vi "Auto_New.vi"() -> ()   [LabVIEW 2023]
uses:
  Control/Saurabh/prosucer_consumer_enum.ctl
  <vilib>/addons/database/NI_Database_API.lvlib
  Global/Global 1.vi
  Global/DATA LOG.vi
  <vilib>/Utility/error.llb/DialogType.ctl
  <vilib>/addons/database/Connection.llb/DB Tools Open Connec (String).vi
panel:
  out "SHIFT":string
  in  "BARCODE RECIPE":string(combo)
  out "PLC COM.":bool
  out "SHIFT_DATA":string[](array[string])
  out "OP40 BARCODE STRING EMPRTY":bool
  out "OP30 BARCODE STRING EMPRTY":bool
  out "stop":bool
  out "error out 2":errorcluster
  out "Shift 4":i32
  out "Time Stamp Out":timestamp[](array[timestamp]) format="%<%X>T"
  out "Time Stamp Out 4":timestamp[](array[timestamp]) format="%<%X>T"
  out "Shift_change":bool
  out "appended array":string[][](array[string])
  out "SHIFT_DATA 2":string[](array[string])
  in  "error in (no error)":errorcluster
  in  "Tab Control":enum32{"Screen 1", "Screen 2"}(tab)
  out "OP 50":bool
  out "OP 40":bool
  out "OP 30":bool
  out "OP - 50":T1
  out "OP - 40":T2
  out "OP - 30":T3
  in  "stop 2":bool
  out "OP - 10":T4
  in  "SIMULATE INPUT":bool[](array[boolean])=[FALSE, FALSE, FALSE, FALSE]
  out "OP - 20":T5
  out "OP 10 & 20":bool
  out "OP - 110":cluster{"BARCODE":string}
  out "OP - 80":T6
  out "OP - 70":T7
  out "OP - 90":T8
  out "OP - 100":T9
  out "OP - 60":T10
  out "OP 60":bool
  out "OP 70 & 80":bool
  out "OP 90 -100 - 110":bool
  # "SENSOR MIN VLTG"
  # "Op10 20\nOp30\nOp 40\nOp50\nOp60\nOp70-80\nOp 90-100-110"
  # "OP - 50"
  # "OP - 40"
  # "OP - 30"
  # "OP - 10"
  # "OP - 20"
  # "Op10 20\nOp30\nOp 40\nOp50\nOp60\nOp70-80\nOp 90-100-110"
  # "OP - 110"
  # "OP - 80"
  # "OP - 70"
  # "OP - 90"
  # "OP - 100"
  # "OP - 60"
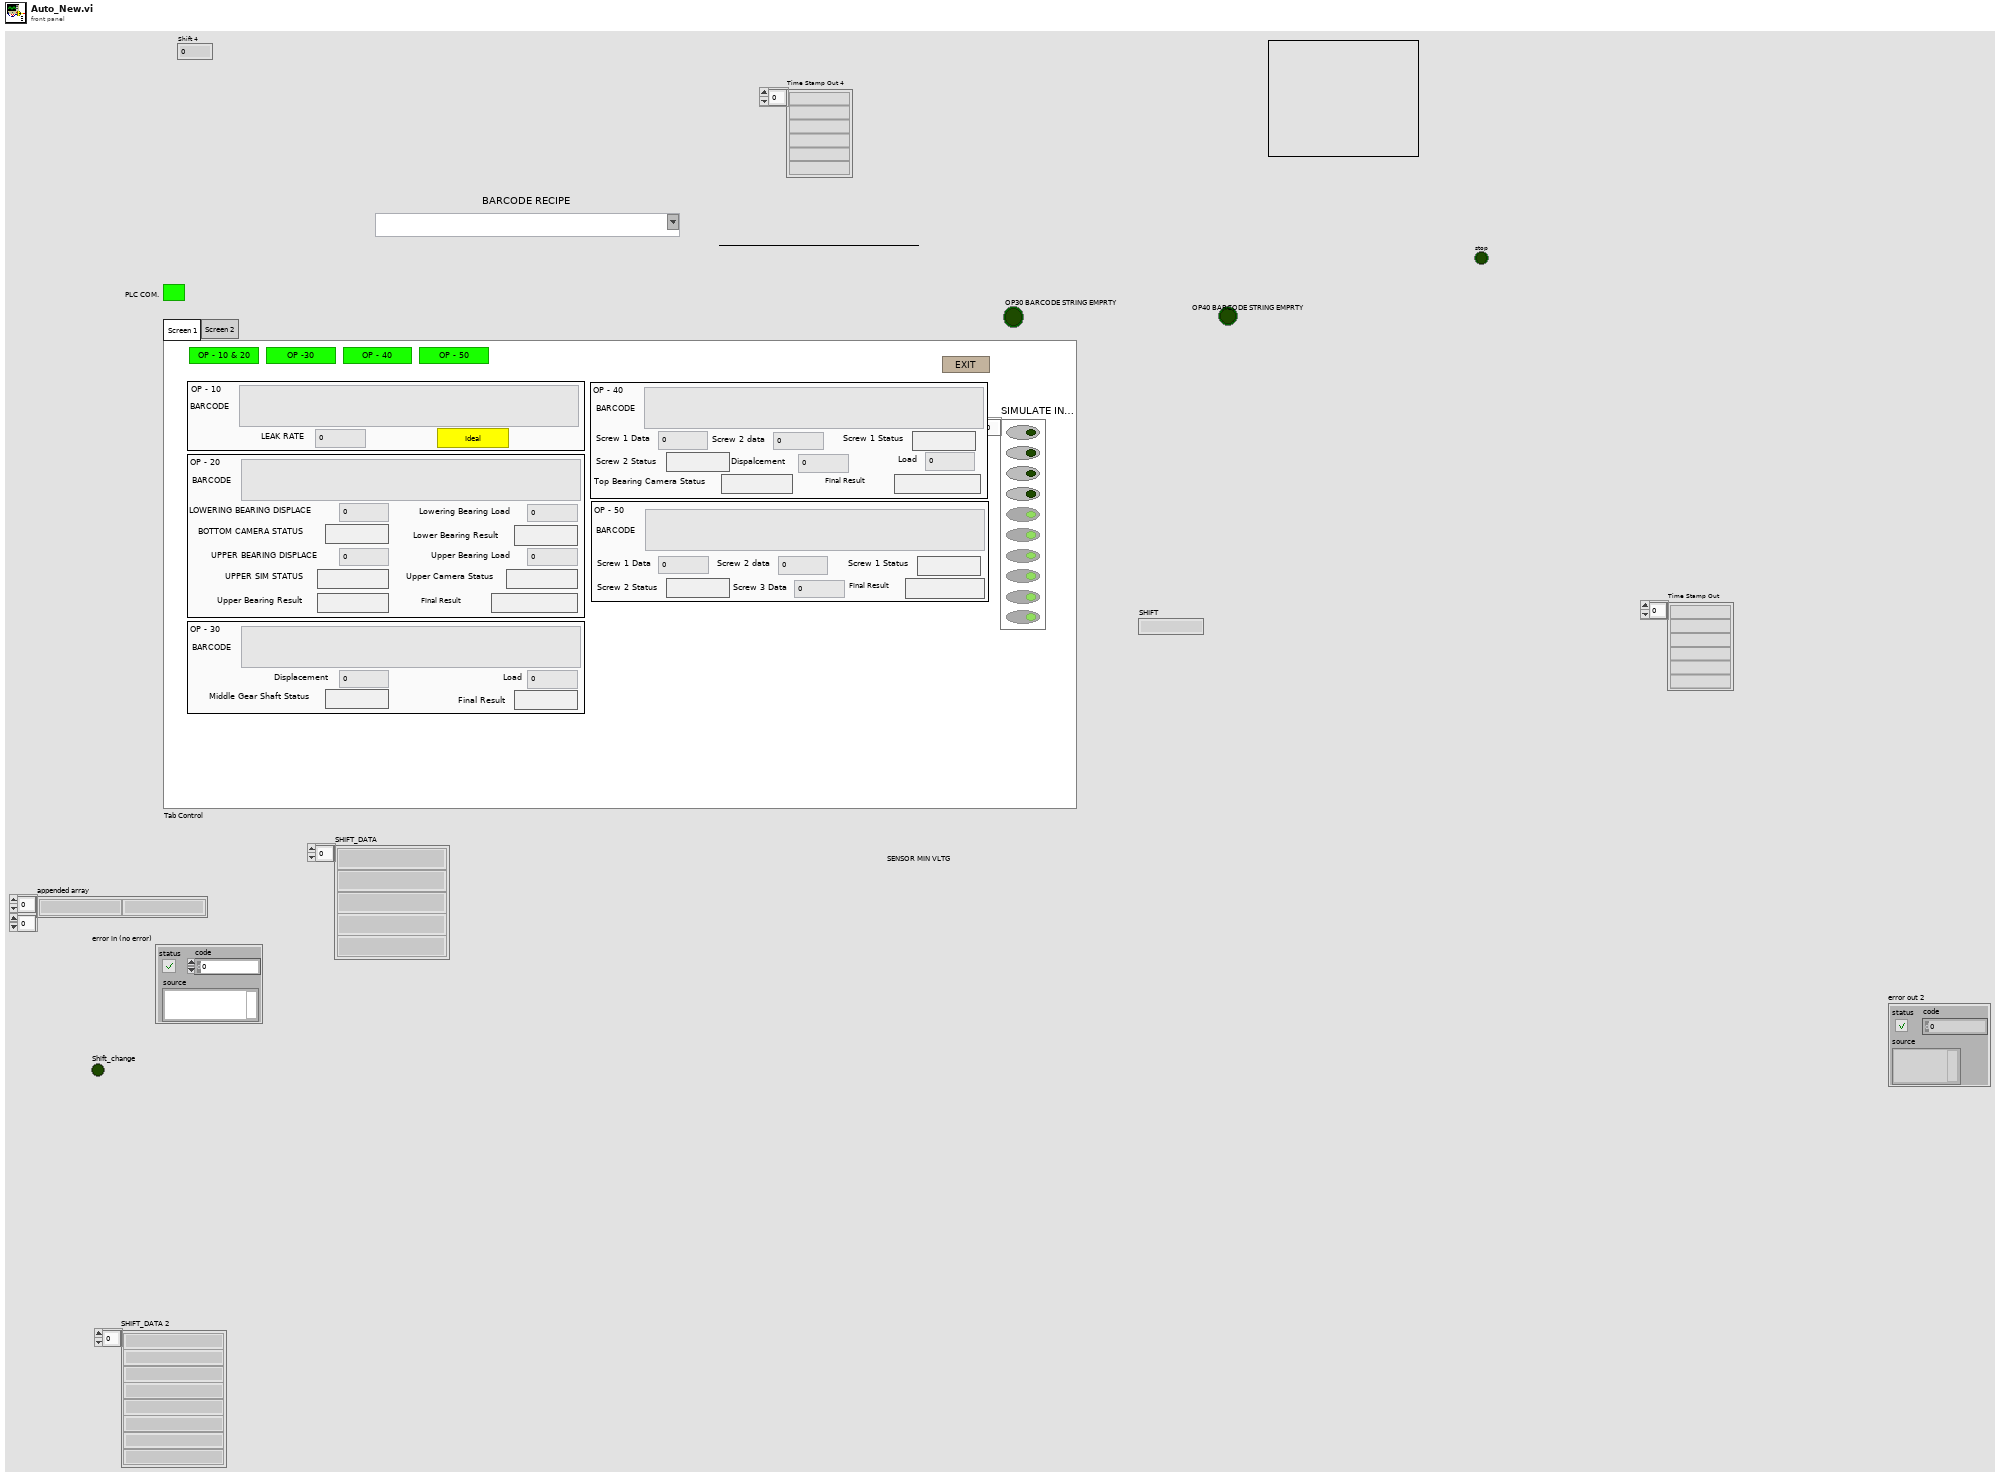
[diagram p1: front panel]
types:
  T1 = cluster{"BARCODE":string, "Screw 1 Data":dbl, "Screw 2 data":dbl, "Screw 1 Status":bool, "Screw 2 Status":bool, "Screw 3 Data":dbl, "Final Result":bool}
  T2 = cluster{"BARCODE":string, "Screw 1 Data":dbl, "Screw 2 data":dbl, "Screw 1 Status":bool, "Screw 2 Status":bool, "Dispalcement ":dbl, "Load ":dbl, "Top Bearing Camera Status":bool, "Final Result":bool}
  T3 = cluster{"BARCODE":string, "Displacement":dbl, "Load":dbl, "Middle Gear Shaft Status":bool, "Final Result":bool}
  T4 = cluster{"BARCODE":string, "LEAK RATE":dbl, "RESULT":bool}
  T5 = cluster{"BARCODE":string, "LOWERING BEARING DISPLACE":dbl, "Lowering Bearing Load":dbl, "BOTTOM CAMERA STATUS":bool, "Lower Bearing Result":bool, "UPPER BEARING DISPLACE":dbl, "Upper Bearing Load ":dbl, "UPPER SIM STATUS":bool, "Upper Camera Status":bool, "Upper Bearing Result":bool, "Final Result":bool}
  T6 = cluster{"BARCODE":string, "Load":dbl, "Final Result":bool, "Dispensing":bool}
  T7 = cluster{"BARCODE":string, "Sensor MIN Vltg":dbl, "Sensor MAX Vltg":dbl, "Final Result":bool}
  T8 = cluster{"BARCODE":string, "Seat LT Data":dbl, "Seat Status":bool, "Steam LT Data":dbl, "Final Result":bool}
  T9 = cluster{"BARCODE":string, "Sensor O/P Open V":dbl, "Start Of Close Sensor V":dbl, "Final Result":bool, "Sensor O/P Full Close V":dbl, "Response Time FWD (mSec)":dbl, "Response Time REV (mSec)":dbl, "Motor V Start Of Close A":dbl, "Motor V Full Close B R":dbl, "Motor V Start Back C":dbl, "Motor V Full Open D":dbl, "Motor RMS Current A":dbl}
  T10 = cluster{"BARCODE":string, "Screw 1 Data":dbl, "Screw 2 data":dbl, "Screw 1 Status":bool, "Screw 2 Status":bool, "Screw3 Data":dbl, "Final Result":bool, "Screw3 Status":bool, "Screw4 Data":dbl, "Screw5 Data":dbl, "Screw4 Status":bool, "Screw5 Status":bool, "Screw6 Data":dbl, "Screw6 Status":bool}
  T11 = cluster{"OP - 10":cluster{"BARCODE":string, "LEAK RATE":dbl, "RESULT":bool}, "OP - 20":cluster{"BARCODE":string, "LOWERING BEARING DISPLACE":dbl, "LOWERING BEARING LOAD":dbl, "BOTTOM CAMERA STATUS":bool, "LOWER BEARING RESULT":bool, "UPPER BEARING DISPLACE":dbl, "UPPER BEARING LOAD ":dbl, "UPPER SIM STATUS":bool, "UPPER CAMERA STATUS":bool, "UPPER BEARING RESULT":bool, "FINAL RESULT":bool}, "OP - 30":cluster{"BARCODE":string, "Displacement":dbl, "Load":dbl, "Middle Gear Shaft Status":bool, "Final Result":bool}, "OP - 40":cluster{"BARCODE":string, "Screw 1 Data":dbl, "Screw 2 data":dbl, "Screw 1 Status":bool, "Screw 2 Status":bool, "Dispalcement ":dbl, "Load ":dbl, "Top Bearing Camera Status":bool, "Final Result":bool}, "OP - 50":cluster{"BARCODE":string, "Screw 1 Data":dbl, "Screw 2 data":dbl, "Screw 1 Status":bool, "Screw 2 Status":bool, "Screw 3 Data":dbl, "Final Result":bool}, "OP - 60":cluster{"BARCODE":string, "Screw 1 Data":dbl, "Screw 2 data":dbl, "Screw 1 Status":bool, "Screw 2 Status":bool, "Screw3 Data":dbl, "Final Result":bool, "Screw3 Status":bool, "Screw4 Data":dbl, "Screw5 Data":dbl, "Screw4 Status":bool, "Screw5 Status":bool, "Screw6 Data":dbl, "Screw6 Status":bool}, "OP - 70":cluster{"BARCODE":string, "Sensor MIN Vltg":dbl, "Sensor MAX Vltg":dbl, "Final Result":bool}, "OP - 80":cluster{"BARCODE":string, "Load":dbl, "Final Result":bool, "Dispensing":bool}, "OP - 90":cluster{"BARCODE":string, "Seat LT Data":dbl, "Seat Status":bool, "Steam LT Data":dbl, "Final Result":bool}, "OP - 100":cluster{"BARCODE":string, "Sensor O/P Open V":dbl, "Start Of Close Sensor V":dbl, "Final Result":bool, "Sensor O/P Full Close V":dbl, "Response Time FWD (mSec)":dbl, "Response Time REV (mSec)":dbl, "Motor V Start Of Close A":dbl, "Motor V Full Close B R":dbl, "Motor V Start Back C":dbl, "Motor V Full Open D":dbl, "Motor RMS Current A":dbl}, "OP - 110":cluster{"BARCODE":string}}
  T12 = typedef "prosucer_consumer_enum.ctl" = enum16{"SCAN1", "SCAN2", "SCAN3", "SCAN4", "SCAN5", "SCAN6", "SCAN7", "SCAN8", "SCAN9", "SCAN10", "SCAN11", "STOP", "DATALOG1", "DATALOG2", "DATALOG3", "DATALOG4", "DATALOG5", "DATALOG6", "DATALOG7", "DATALOG8", "DATALOG9", "DATALOG10", "DATALOG11", "-1", "CYCLE_START1", "CYCLE_START2", "CYCLE_START3", "CYCLE_START4", "BARCODE RECIPE", "EMERGENCY STOP"}
  T13 = typedef "NI_Database_API.lvlib/Conn ObjectReference.ctl" = refnum<k1>
  T14 = typedef "DialogType.ctl" = u16
  T15 = cluster{"trimmed string":string, "SHIFT":string, "date/time string":string, string, "Input 2":string}
  T16 = cluster{"SHIFT":string, "date/time string":string, "Input 2":string}
  T17 = cluster{"Input 2":string, "Input 2":string, "Input 2":string, "Input 2":string, "Input 2":string, "Input 2":string, "Input 2":string, "Input 2":string, "Input 2":string, "Input 2":string}
  T18 = cluster{"SHIFT":string, "date/time string":string, void}
  T19 = cluster{"BARCODE":string, "LOWERING BEARING DISPLACE":dbl, "LOWERING BEARING LOAD":dbl, "BOTTOM CAMERA STATUS":bool, "LOWER BEARING RESULT":bool, "UPPER BEARING DISPLACE":dbl, "UPPER BEARING LOAD ":dbl, "UPPER SIM STATUS":bool, "UPPER CAMERA STATUS":bool, "UPPER BEARING RESULT":bool, "FINAL RESULT":bool}
  T20 = enum32{"invalid app kind", "Development System", "Run Time System", "Student Edition", "Embedded LabVIEW", "Evaluation", "Custom"}
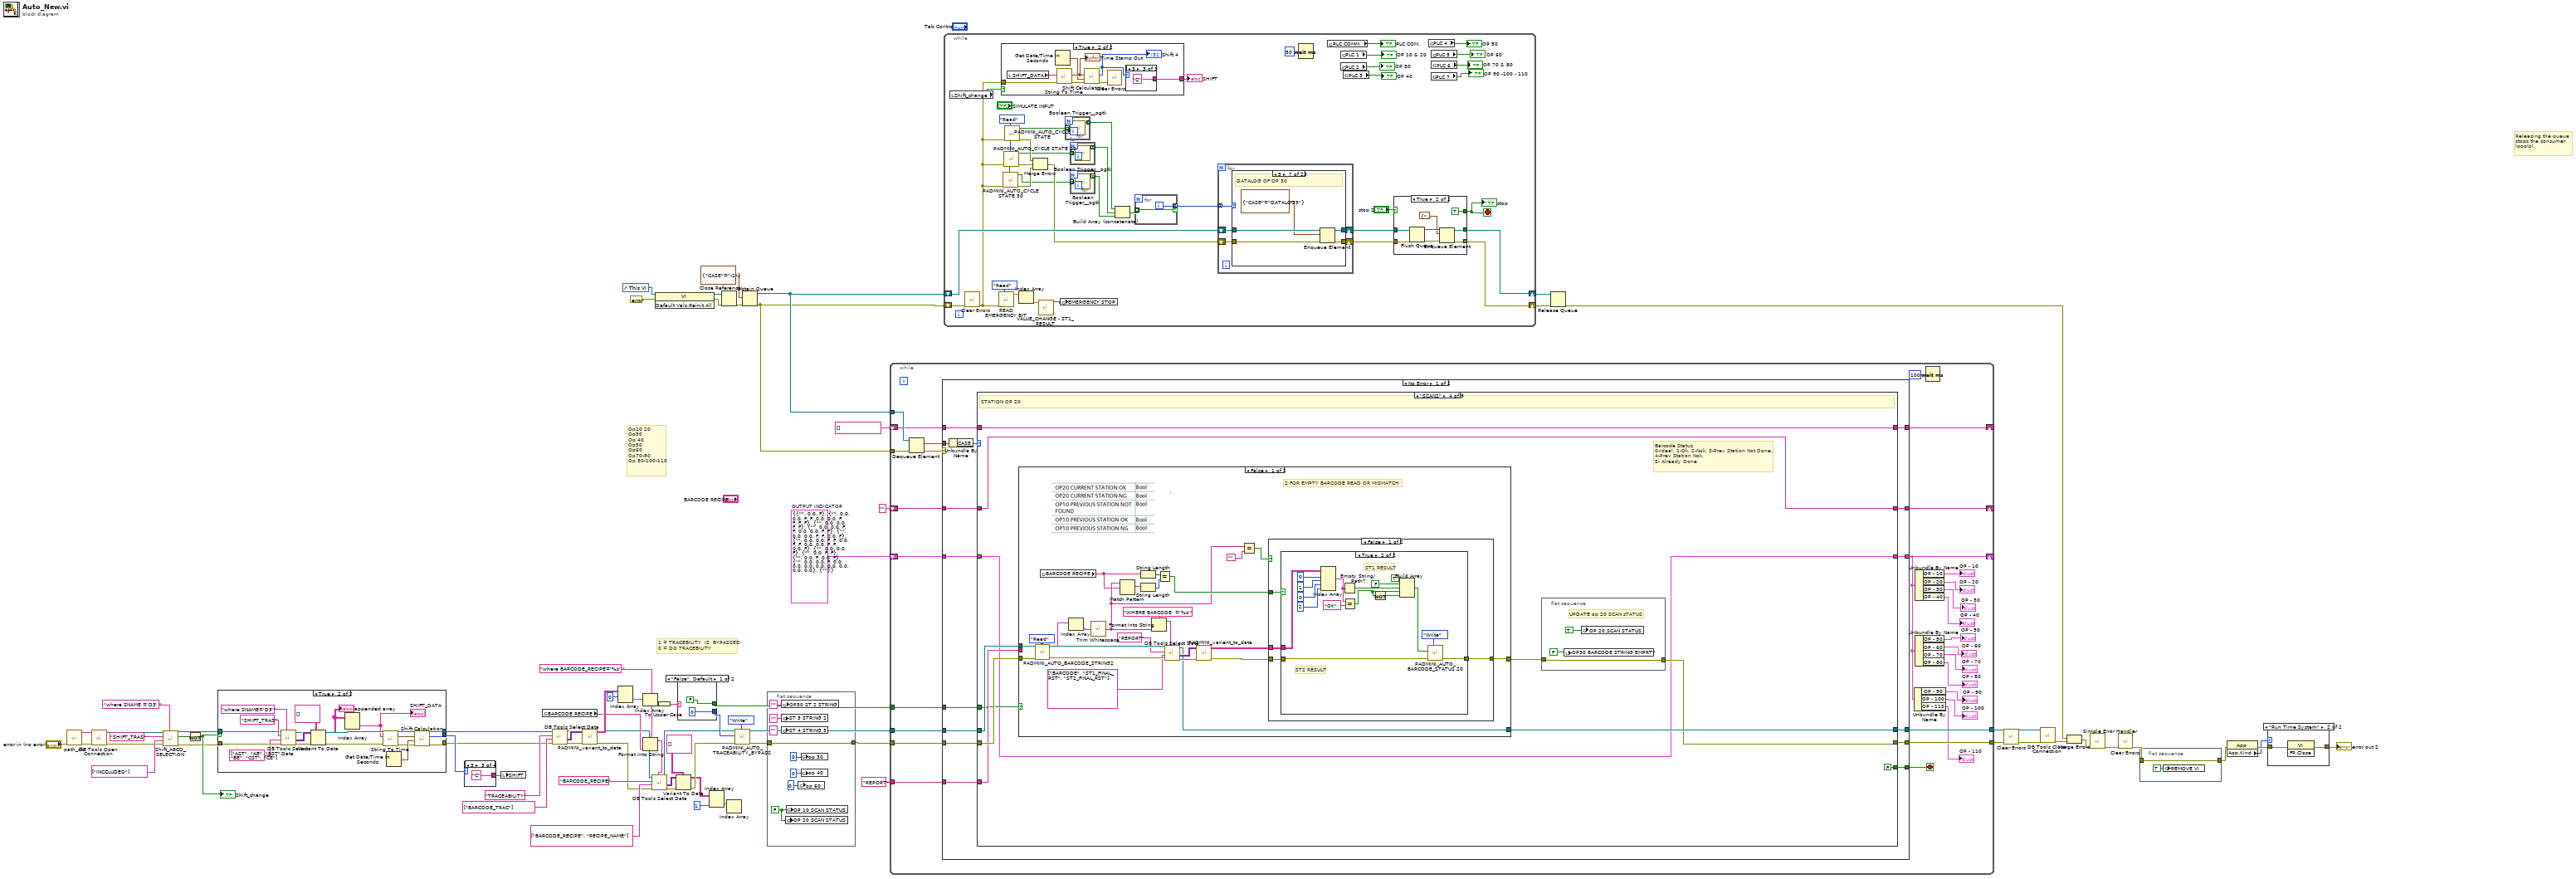
[diagram p0: block diagram]
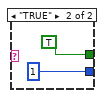
[diagram p2: hidden frame]
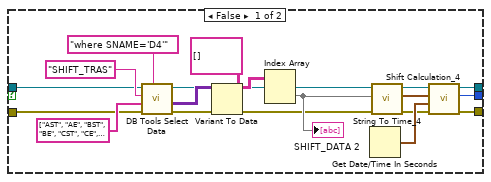
[diagram p3: hidden frame]
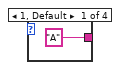
[diagram p4: hidden frame]
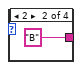
[diagram p5: hidden frame]
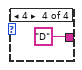
[diagram p6: hidden frame]
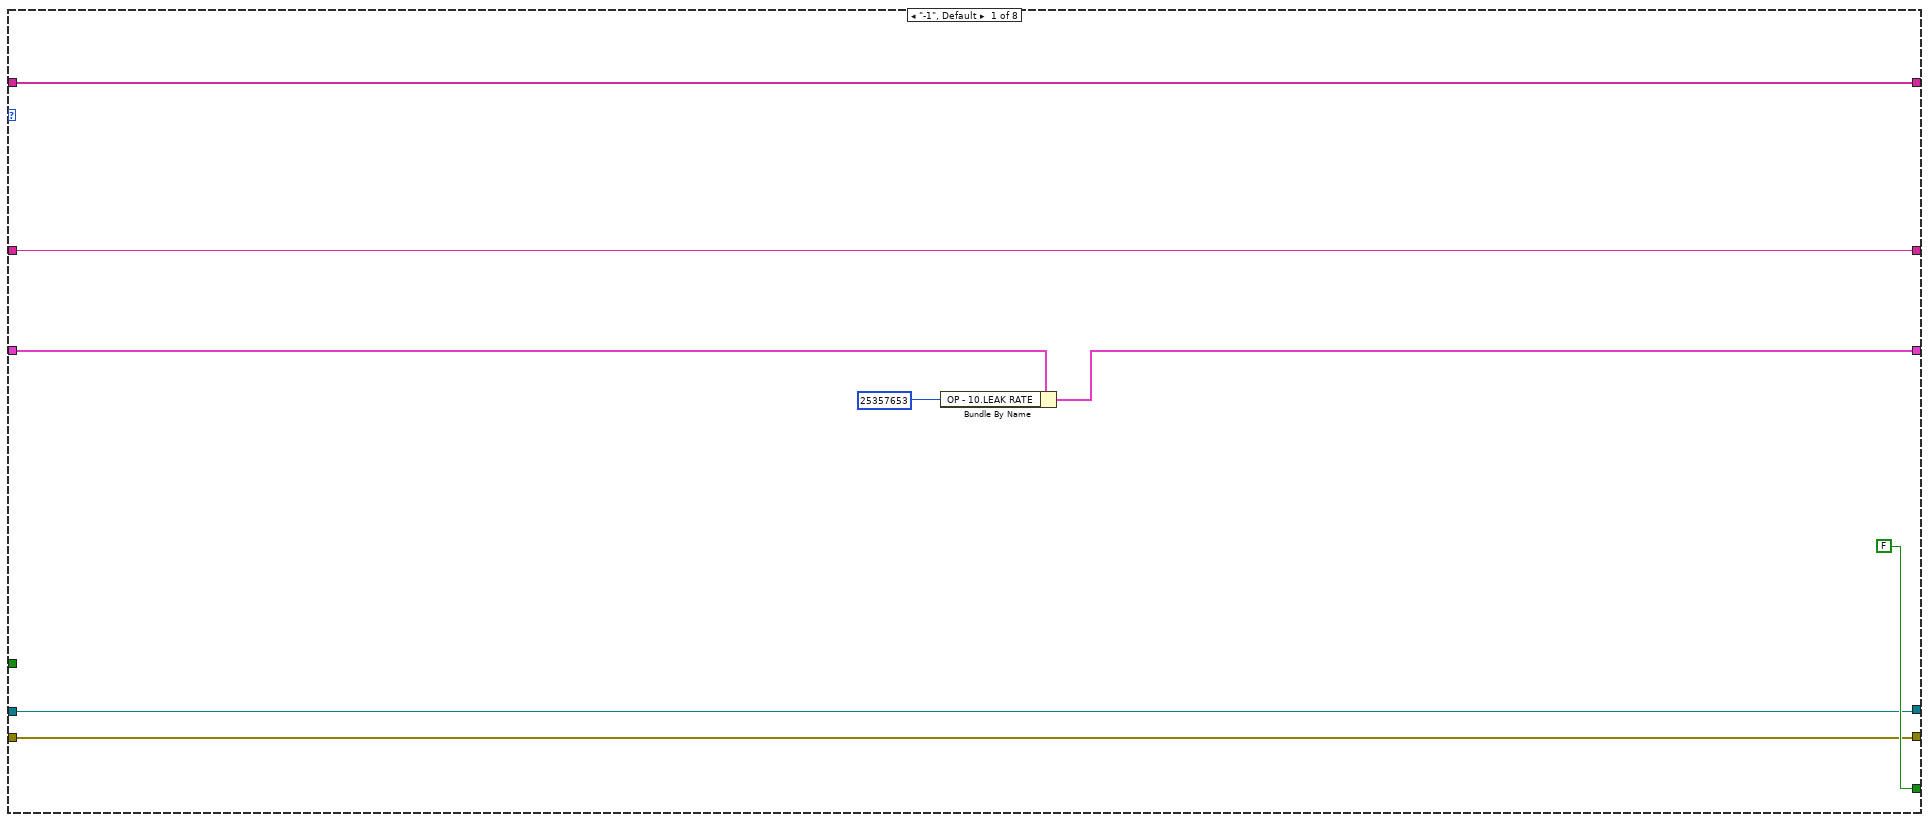
[diagram p7: hidden frame]
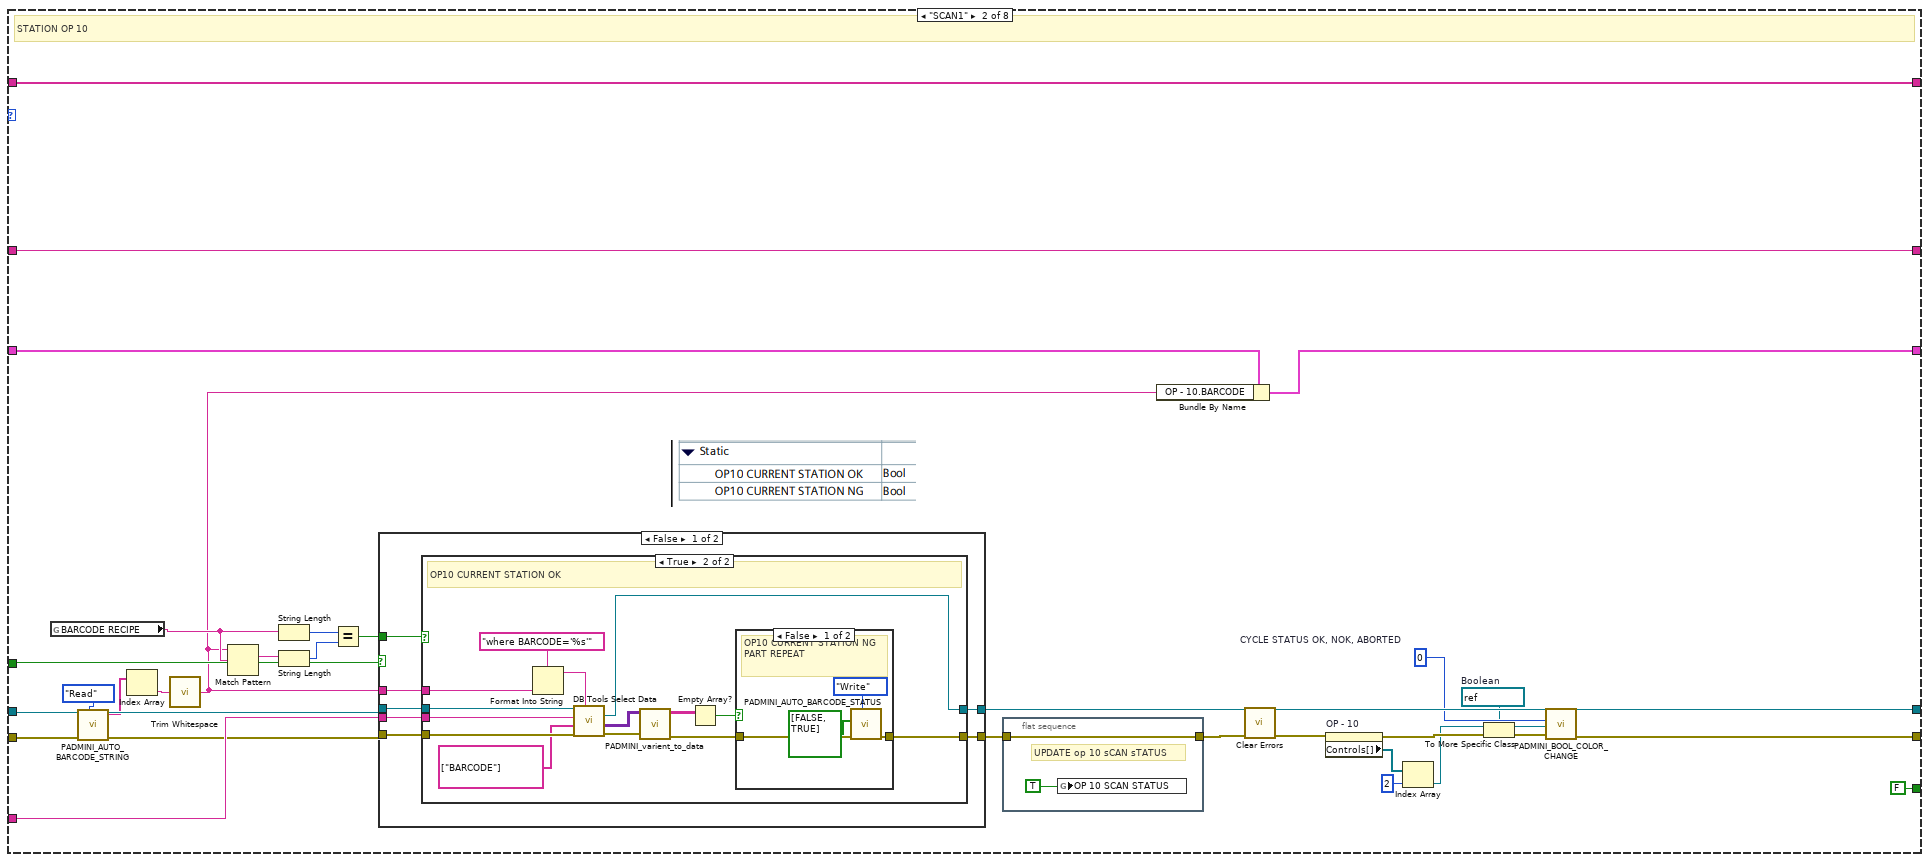
[diagram p8: hidden frame]
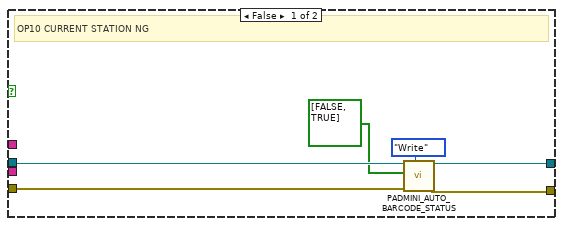
[diagram p9: hidden frame]
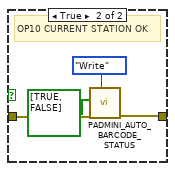
[diagram p10: hidden frame]
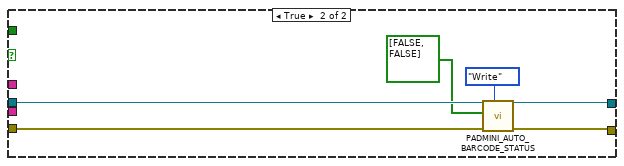
[diagram p11: hidden frame]
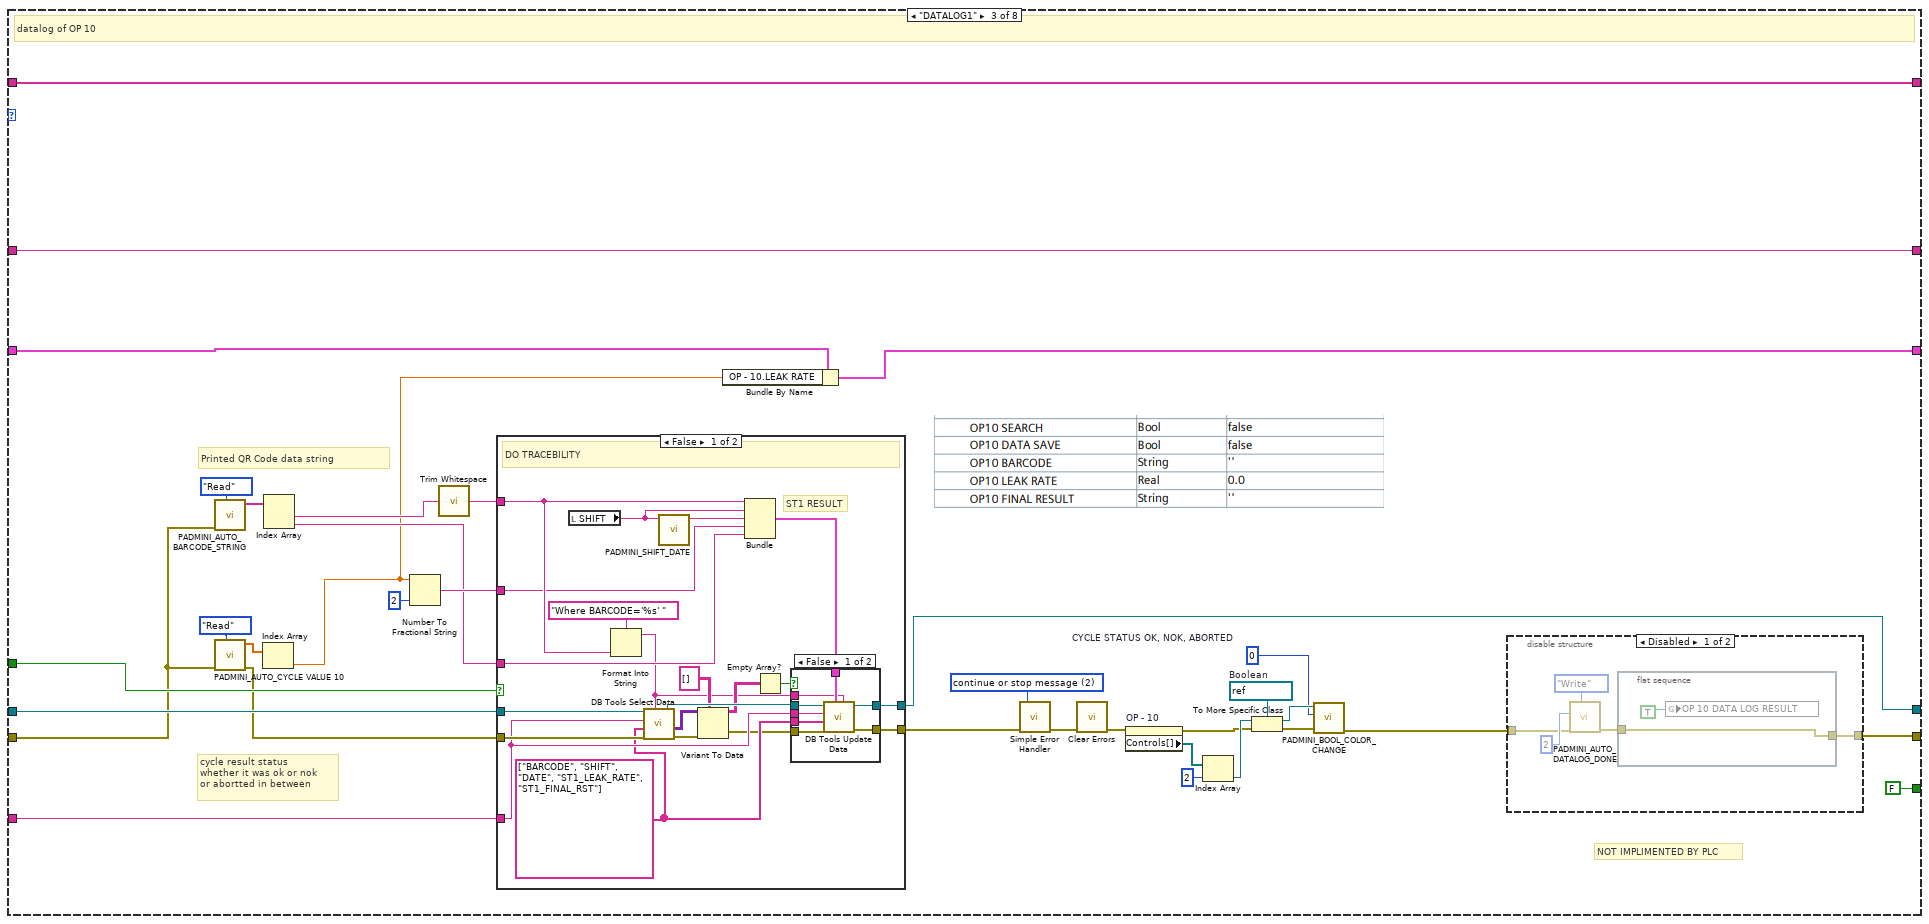
[diagram p12: hidden frame]
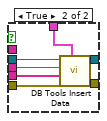
[diagram p14: hidden frame]
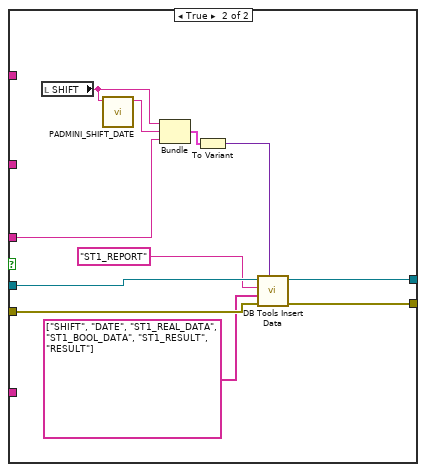
[diagram p15: hidden frame]
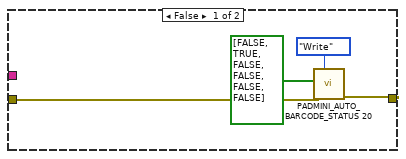
[diagram p16: hidden frame]
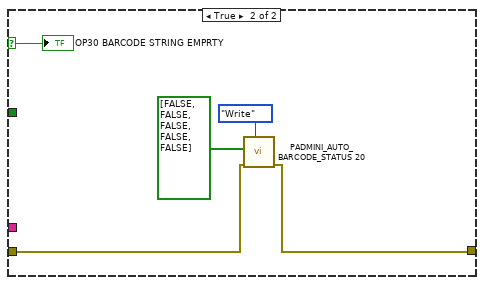
[diagram p17: hidden frame]
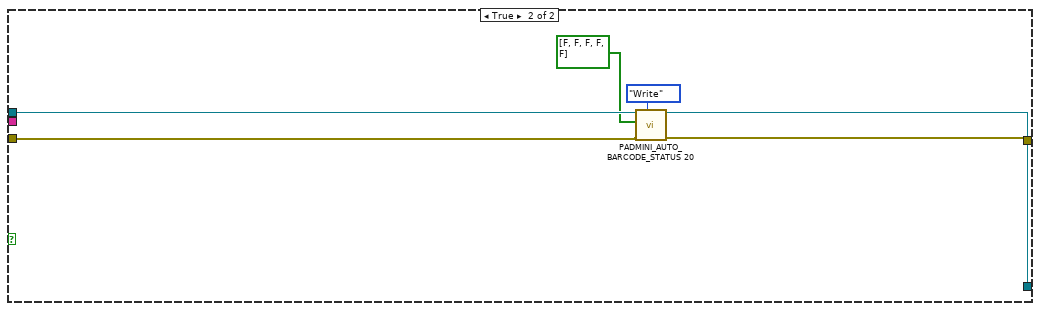
[diagram p18: hidden frame]
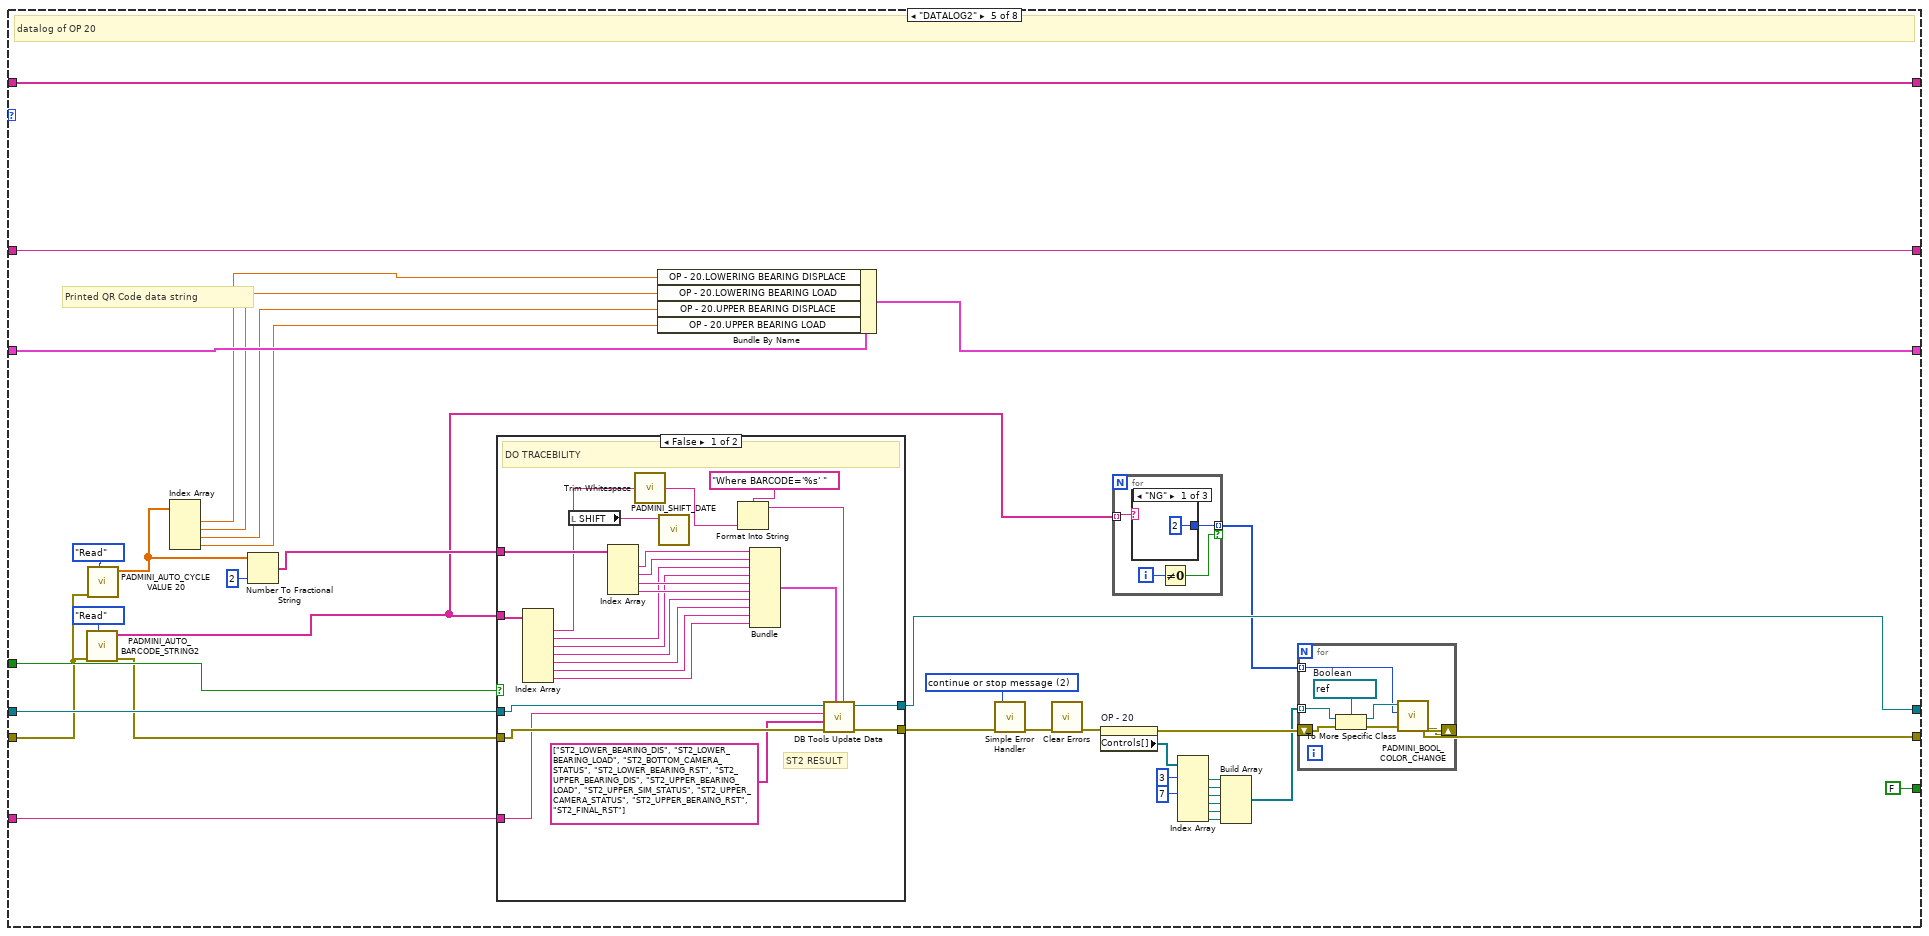
[diagram p19: hidden frame]
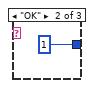
[diagram p20: hidden frame]
diagram:
  w2 = T11 {"OP - 10"={"BARCODE"="", "LEAK RATE"=0.0, "RESULT"=FALSE}, "OP - 20"={"BARCODE"="", "LOWERING BEARING DISPLACE"=0.0, "LOWERING BEARING LOAD"=0.0, "BOTTOM CAMERA STATUS"=FALSE, "LOWER BEARING RESULT"=FALSE, "UPPER BEARING DISPLACE"=0.0, "UPPER BEARING LOAD "=0.0, "UPPER SIM STATUS"=FALSE, "UPPER CAMERA STATUS"=FALSE, "UPPER BEARING RESULT"=FALSE, "FINAL RESULT"=FALSE}, "OP - 30"={"BARCODE"="", "Displacement"=0.0, "Load"=0.0, "Middle Gear Shaft Status"=FALSE, "Final Result"=FALSE}, "OP - 40"={"BARCODE"="", "Screw 1 Data"=0.0, "Screw 2 data"=0.0, "Screw 1 Status"=FALSE, "Screw 2 Status"=FALSE, "Dispalcement "=0.0, "Load "=0.0, "Top Bearing Camera Status"=FALSE, "Final Result"=FALSE}, "OP - 50"={"BARCODE"="", "Screw 1 Data"=0.0, "Screw 2 data"=0.0, "Screw 1 Status"=FALSE, "Screw 2 Status"=FALSE, "Screw 3 Data"=0.0, "Final Result"=FALSE}, "OP - 60"={"BARCODE"="", "Screw 1 Data"=0.0, "Screw 2 data"=0.0, "Screw 1 Status"=FALSE, "Screw 2 Status"=FALSE, "Screw3 Data"=0.0, "Final Result"=FALSE, "Screw3 Status"=FALSE, "Screw4 Data"=0.0, "Screw5 Data"=0.0, "Screw4 Status"=FALSE, "Screw5 Status"=FALSE, "Screw6 Data"=0.0, "Screw6 Status"=FALSE}, "OP - 70"={"BARCODE"="", "Sensor MIN Vltg"=0.0, "Sensor MAX Vltg"=0.0, "Final Result"=FALSE}, "OP - 80"={"BARCODE"="", "Load"=0.0, "Final Result"=FALSE, "Dispensing"=FALSE}, "OP - 90"={"BARCODE"="", "Seat LT Data"=0.0, "Seat Status"=FALSE, "Steam LT Data"=0.0, "Final Result"=FALSE}, "OP - 100"={"BARCODE"="", "Sensor O/P Open V"=0.0, "Start Of Close Sensor V"=0.0, "Final Result"=FALSE, "Sensor O/P Full Close V"=0.0, "Response Time FWD (mSec)"=0.0, "Response Time REV (mSec)"=0.0, "Motor V Start Of Close A"=0.0, "Motor V Full Close B R"=0.0, "Motor V Start Back C"=0.0, "Motor V Full Open D"=0.0, "Motor RMS Current A"=0.0}, "OP - 110"={"BARCODE"=""}}  # OUTPUT INDICATOR
  # "Op10 20\nOp30\nOp 40\nOp50\nOp60\nOp70-80\nOp 90-100-110"
  # "1 = TRACEBILITY  IS  BYPASSED\n0 = DO TRACEBILITY"
  # "Releasing the queue stops the consumer loop(s)."
  n1 = call "path_db.vi"("error in"="error in (no error)") -> ("error out"=w47:errorcluster, "resulting string"=w68:string)  [unwired: 9 in]
  n2 = call-poly <vilib>:"DB Tools Open Connection.vi"("error in (no error)"=w47, "connection information"=w68) -> ("error out"=w46:errorcluster, "connection reference"=w39:T13)  [unwired: 6 in]
  n3 = call "Shift_ABCD_SELECTION.vi"("Where"="where SNAME ='D3' ", "error in (no error)"=w46, "Array"=string[] ["INCCLUDED"], "table"="SHIFT_TRAS", "Refnum in"=w39) -> ("error out"=w1:errorcluster, "Boolean"=w59:bool, "Refnum out"=w60:T13)  [unwired: 4 in]
  n4 = Not(x=w59) -> (.not. x?=w58:bool)
  "Shift_change" <- w58
  n5 = case shown="True" w58 {
    tunnel: [w73 w97] -> w64
    tunnel: w60 -> [w76 w95]
    tunnel: w1 -> [w75 w94]
    tunnel: [w74 w93] -> w28
    tunnel: [w72 w87] -> w27
    frame False {
      n6 = call <vilib>:"DB Tools Select Data.vi"("condition"="where SNAME='D4'", "error in (no error)"=w75, "columns"=string[] ["AST", "AE", "BST", "BE", "CST", "CE", "DST", "DE"], "table"="SHIFT_TRAS", "connection reference"=w76) -> ("error out"=w82:errorcluster, "data"=w86:variant[][], "connection reference out"=w74:T13)  [unwired: 1 in]
      n7 = Variant To Data(error in=w82, type=string[][] [], Variant=w86) -> (data=w79:string[][], error out=w72:errorcluster)
      n8 = Index Array(array=w79) -> (element=w78:string[])  [unwired: 2 in]
      "SHIFT_DATA 2" <- w78
      n9 = Get Date/Time In Seconds() -> (seconds since 1Jan1904=w81:timestamp)
      n10 = call "String To Time_4.vi"("String Array In"=w78) -> ("Time Stamp Out"=w77:timestamp[])  [unwired: 9 in, 1 out]
      n11 = call "Shift Calculation_4.vi"("Current Time"=w81, "Time Stamp Out"=w77) -> ("Shift"=w73:i32)  [unwired: 8 in, 1 out]
    }
    frame True {
      n12 = call <vilib>:"DB Tools Select Data.vi"("condition"="where SNAME='D3'", "error in (no error)"=w94, "columns"=string[] ["AST", "AE", "BST", "BE", "CST", "CE"], "table"="SHIFT_TRAS", "connection reference"=w95) -> ("error out"=w99:errorcluster, "data"=w103:variant[][], "connection reference out"=w93:T13)  [unwired: 1 in]
      n13 = Variant To Data(error in=w99, type=string[][] [], Variant=w103) -> (data=w91:string[][], error out=w89:errorcluster)
      "appended array" <- w91
      n14 = Index Array(array=w91) -> (element=w90:string[])  [unwired: 2 in]
      "SHIFT_DATA" <- w90
      n15 = call "String To Time.vi"("error in (no error)"=w89, "String Array In"=w90) -> ("error out"=w88:errorcluster, "Time Stamp Out"=w96:timestamp[])  [unwired: 8 in]
      n16 = Get Date/Time In Seconds() -> (seconds since 1Jan1904=w98:timestamp)
      n17 = call "Shift Calculation.vi"("error in (no error)"=w88, "Current Time"=w98, "Time Stamp Out"=w96) -> ("error out"=w87:errorcluster, "Shift"=w97:i32)  [unwired: 7 in]
    }
  }
  n18 = case shown="3" w64 {
    tunnel: ["A" "B" "C" "D"] -> w57
    frame 1, Default {
    }
    frame 2 {
    }
    frame 3 {
    }
    frame 4 {
    }
  }
  n19 = local write "SHIFT"(w57) -> ()
  n20 = global read "Global 1.vi" "BARCODE RECIPE"() -> (w8:string)
  n21 = call <vilib>:"DB Tools Select Data.vi"("error in (no error)"=w27, "columns"=string[] ["BARCODE_TRAC"], "table"="TRACEABILITY", "connection reference"=w28) -> ("error out"=w37:errorcluster, "data"=w36:variant[][], "connection reference out"=w14:T13)  [unwired: 2 in]
  n22 = call "PADMINI_varient_to_data.vi"("error in (no error)"=w37, "data"=w36) -> ("error out"=w12:errorcluster, "Array"=w35:string[][])  [unwired: 8 in]
  n23 = Index Array(array=w35, index (row)=0 ("disabled index (col)")) -> (element=w34:string[])  [unwired: 1 in]
  n24 = control-ref of="This VI"() -> (w44:refnum<vi>)
  n25 = Index Array(array=w34) -> (element=w30:string)  [unwired: 1 in]
  n26 = Format Into String(format string="where BARCODE_RECIPE='%s' ", w8) -> (resulting string=w6:string)  [unwired: 2 in, 1 out]
  n27 = call <vilib>:"DB Tools Select Data.vi"("condition"=w6, "error in (no error)"=w12, "columns"=string[] ["BARCODE_RECIPE", "RECIPE_NAME"], "table"="BARCODE_RECIPE", "connection reference"=w14) -> ("error out"=w16:errorcluster, "data"=w15:variant[][], "connection reference out"=w13:T13)  [unwired: 1 in]
  n28 = invoke class="VI" method="Default Vals.Reinit All"(reference=w44, error in=errorcluster {"status"=FALSE, "code"=0, "source"=""} ("error in (no error)")) -> (reference out=w42:refnum<vi>, error out=w43:errorcluster)  [unwired: 1 in, 1 out]
  n29 = To Upper Case(1:w30) -> (0:w29:string)
  n30 = Variant To Data(error in=w16, type=string[][] [], Variant=w15) -> (data=w9:string[][], error out=w11:errorcluster)
  n31 = case shown="\"False\", Default" w29 {
    tunnel: [FALSE ("BARCODE TRACEABILITY") TRUE ("BARCODE TRACEABILITY")] -> w19
    tunnel: [0 1] -> w25
    frame "False", Default {
    }
    frame "TRUE" {
    }
  }
  n32 = Index Array(array=w9, index (col)=1 ("disabled index (col)")) -> (element=w4:string[])  [unwired: 1 in]
  n33 = Close Reference(reference=w42, error in (no error)=w43) -> (error out=w40:errorcluster)
  n34 = Index Array(array=w4) -> ()  [unwired: 1 in, 1 out]
  n35 = call "PADMINI_AUTO_TRACEABILITY_BYPASS.vi"("Enum"=enum16{"Read", "Write"}."Write", "error in (no error)"=w11, "I/P"=w25) -> ("error out"=w23:errorcluster)  [unwired: 7 in, 1 out]
  n36 = Obtain Queue(element data type=cluster{"CASE":T12} {"CASE"=enum."-1"}, error in (no error)=w40) -> (queue out=w69:refnum<queue>, error out=w20:errorcluster)  [unwired: 3 in, 1 out]
  n37 = flat-sequence {
    tunnel: w23 -> [w116]
    tunnel: [w116] -> w22
    frame #0 {
      w112 = FALSE
      n38 = global write "DATA LOG.vi" "ST 3 STRING 2"("" ("ST 3 STRING 2")) -> ()
      n39 = global write "DATA LOG.vi" "ST 4 STRING 3"("" ("ST 4 STRING 3")) -> ()
      n40 = global write "DATA LOG.vi" "OP30 ST 2 STRING"("" ("OP30 ST 2 STRING")) -> ()
      n41 = global write "DATA LOG.vi" "OP 20 SCAN STATUS"(w112) -> ()
      n42 = global write "DATA LOG.vi" "OP 10 SCAN STATUS"(w112) -> ()
      n43 = global write "DATA LOG.vi" "op 60"(0 ("op 30")) -> ()
      n44 = global write "DATA LOG.vi" "op 30"(0 ("op 30")) -> ()
      n45 = global write "DATA LOG.vi" "op 40"(0 ("op 30")) -> ()
    }
  }
  n46 = while {
    tunnel: w69 -> [w148]
    tunnel: w20 -> [w144]
    tunnel: w22 -> [w143]
    tunnel: w13 -> [w142]
    tunnel: [w141] -> w67
    tunnel: [w140] -> w66
    tunnel: w19 -> [w139]
    tunnel: "REPORT" -> [w138]
    shift-right: [w136] -> _
    shift-left: string[] [] -> [w137]
    shift-right: [w135] -> _
    shift-left: "" ("trimmed string") -> [w134]
    shift-right: [w123] -> _
    shift-left: w2 -> [w132]
    stop <- w145 stop-if-true
    n47 = Dequeue Element(queue=w148, error in (no error)=w144) -> (element=w146:cluster{"CASE":T12}, error out=w147:errorcluster)  [unwired: 1 in, 2 out]
    n48 = case shown="No Error" w147 {
      tunnel: w146 -> [w163 _]
      tunnel: [w159 TRUE] -> w145
      tunnel: w143 -> [w160 w643]
      tunnel: w142 -> [w161 w642]
      tunnel: [w157 w643] -> w141
      tunnel: [w158 w642] -> w140
      tunnel: w139 -> [w156 _]
      tunnel: w138 -> [w155 _]
      tunnel: w137 -> [w154 w641]
      tunnel: [w153 w641] -> w136
      tunnel: [w152 w640] -> w135
      tunnel: w134 -> [w151 w640]
      tunnel: w132 -> [w150 w639]
      tunnel: [w149 w639] -> w123
      frame No Error {
        n49 = Unbundle By Name(w163) -> ("CASE"=w162:T12)
        n50 = case shown="\"SCAN2\"" w162 {
          tunnel: w161 -> [w170 w202 w278 w345 w443 w506 w626 w634]
          tunnel: w160 -> [w169 w198 w245 w344 w424 w505 w625 w636]
          tunnel: [FALSE FALSE FALSE FALSE FALSE FALSE FALSE TRUE] -> w159
          tunnel: [w170 w200 w275 w342 w440 w503 w626 w633] -> w158
          tunnel: [w169 w177 w274 w339 w430 w500 w625 w635] -> w157
          tunnel: w156 -> [_ w195 w277 w341 w442 w502 _ _]
          tunnel: w155 -> [_ w201 w276 w343 w441 w504 _ _]
          tunnel: w154 -> [w168 w199 w271 w337 w439 w499 w623 w637]
          tunnel: [w168 w199 w271 w337 w439 w499 w623 w637] -> w153
          tunnel: [w167 w194 w267 w336 w435 w498 w622 w628] -> w152
          tunnel: w151 -> [w167 w194 w267 w336 w435 w498 w622 w628]
          tunnel: w150 -> [w166 w188 w256 w335 w429 w497 w621 w627]
          tunnel: [w165 w187 w255 w335 w428 w497 w621 w627] -> w149
          frame "-1", Default {
            n51 = Bundle By Name(cluster=w166, "OP - 10.LEAK RATE"=25357653) -> (w165:T11)
          }
          frame "SCAN1" {
            w180 = u16 0  # CYCLE STATUS OK, NOK, ABORTED
            w179 = refnum<vi> refnum  # Boolean
            # "STATION OP 10"
            n52 = global read "Global 1.vi" "BARCODE RECIPE"() -> (w189:string)
            n53 = call "PADMINI_AUTO_BARCODE_STRING.vi"("Enum"=enum16{"Read", "Write"}."Read", "error in (no error)"=w198) -> ("error out"=w197:errorcluster, "Input 2"=w174:string[])  [unwired: 8 in]
            n54 = Index Array(array=w174) -> (element=w173:string)  [unwired: 1 in]
            n55 = call <vilib>:"Trim Whitespace.vi"("string"=w173) -> ("trimmed string"=w172:string)  [unwired: 1 in]
            n56 = Match Pattern(string=w172, regular expression=w189) -> (match substring=w192:string)  [unwired: 1 in, 3 out]
            n57 = String Length(string=w189) -> (length=w191:i32)
            n58 = String Length(string=w192) -> (length=w190:i32)
            n59 = Equal?(x=w191, y=w190) -> (x = y?=w196:bool)
            n60 = case shown="False" w195 {
              tunnel: w202 -> [w212 w244]
              tunnel: w197 -> [w211 w242]
              tunnel: w201 -> [w210 _]
              tunnel: [w209 w241] -> w176
              tunnel: [w208 w244] -> w200
              tunnel: w196 -> [w207 _]
              tunnel: w172 -> [w206 _]
              frame False {
                n61 = case shown="True" w207 {
                  tunnel: w212 -> [w214 w231]
                  tunnel: w211 -> [w216 w230]
                  tunnel: w210 -> [_ w229]
                  tunnel: [w215 w220] -> w209
                  tunnel: [w214 w219] -> w208
                  tunnel: w206 -> [_ w218]
                  frame False {
                    # "OP10 CURRENT STATION NG"
                    n62 = call "PADMINI_AUTO_BARCODE_STATUS.vi"("Enum"=enum16{"Read", "Write"}."Write", "error in (no error)"=w216, "I/P"=bool[] [FALSE, TRUE]) -> ("error out"=w215:errorcluster)  [unwired: 7 in, 1 out]
                  }
                  frame True {
                    # "OP10 CURRENT STATION OK"
                    n63 = Format Into String(format string="where BARCODE='%s'", w218) -> (resulting string=w226:string)  [unwired: 2 in, 1 out]
                    n64 = call <vilib>:"DB Tools Select Data.vi"("condition"=w226, "error in (no error)"=w230, "columns"=string[] ["BARCODE"], "table"=w229, "connection reference"=w231) -> ("error out"=w225:errorcluster, "data"=w224:variant[][], "connection reference out"=w219:T13)  [unwired: 1 in]
                    n65 = call "PADMINI_varient_to_data.vi"("error in (no error)"=w225, "data"=w224) -> ("error out"=w221:errorcluster, "Array"=w223:string[][])  [unwired: 8 in]
                    n66 = Empty Array?(array=w223) -> (empty?=w222:bool)
                    n67 = case shown="False" w222 {
                      tunnel: w221 -> [w235 w239]
                      tunnel: [w234 w237] -> w220
                      frame False {
                        # "OP10 CURRENT STATION NG\nPART REPEAT"
                        n68 = call "PADMINI_AUTO_BARCODE_STATUS.vi"("Enum"=enum16{"Read", "Write"}."Write", "error in (no error)"=w235, "I/P"=bool[] [FALSE, TRUE]) -> ("error out"=w234:errorcluster)  [unwired: 7 in, 1 out]
                      }
                      frame True {
                        # "OP10 CURRENT STATION OK"
                        n69 = call "PADMINI_AUTO_BARCODE_STATUS.vi"("Enum"=enum16{"Read", "Write"}."Write", "error in (no error)"=w239, "I/P"=bool[] [TRUE, FALSE]) -> ("error out"=w237:errorcluster)  [unwired: 7 in, 1 out]
                      }
                    }
                  }
                }
              }
              frame True {
                n70 = call "PADMINI_AUTO_BARCODE_STATUS.vi"("Enum"=enum16{"Read", "Write"}."Write", "error in (no error)"=w242, "I/P"=bool[] [FALSE, FALSE]) -> ("error out"=w241:errorcluster)  [unwired: 7 in, 1 out]
              }
            }
            n71 = flat-sequence {
              tunnel: [w205] -> w175
              tunnel: w176 -> [w205]
              frame #0 {
                # "UPDATE op 10 sCAN sTATUS"
                n72 = global write "DATA LOG.vi" "OP 10 SCAN STATUS"(TRUE) -> ()
              }
            }
            n73 = Bundle By Name(cluster=w188, "OP - 10.BARCODE"=w172) -> (w187:T11)
            n74 = call <vilib>:"Clear Errors.vi"("error in (no error)"=w175) -> ("error out"=w181:errorcluster)  [unwired: 5 in, 1 out]
            n75 = property on="OP - 10" class="Clust"(error in=w181) -> (error out=w185:errorcluster, "Controls[]"=w183:refnum<vi>[])  [unwired: 1 in, 1 out]
            n76 = Index Array(array=w183, index=2) -> (element=w184:refnum<vi>)
            n77 = To More Specific Class(target class=w179, reference=w184, error in=w185) -> (specific class reference=w182:refnum<vi>, error out=w186:errorcluster)
            n78 = call "PADMINI_BOOL_COLOR_CHANGE.vi"("error in (no error)"=w186, "Numeric"=w180, "Boolean in"=w182) -> ("error out"=w177:errorcluster)  [unwired: 8 in]
          }
          frame "DATALOG1" {
            w257 = u16 0  # CYCLE STATUS OK, NOK, ABORTED
            w261 = refnum<vi> refnum  # Boolean
            w269 = T14 2 items=["no dialog", "OK message", "continue or stop message", "OK message + warnings", "continue/stop + warnings"] ("type of dialog (OK msg:1)")
            # "NOT IMPLIMENTED BY PLC"
            # "cycle result status\nwhether it was ok or nok\nor abortted in between"
            # "Printed QR Code data string"
            # "datalog of OP 10"
            n79 = call "PADMINI_AUTO_BARCODE_STRING.vi"("Enum"=enum16{"Read", "Write"}."Read", "error in (no error)"=w245) -> ("Input 2"=w252:string[])  [unwired: 8 in, 1 out]
            n80 = call "PADMINI_AUTO_CYCLE VALUE 10.vi"("Enum"=enum16{"Read", "Write"}."Read", "error in (no error)"=w245) -> ("error out"=w248:errorcluster, "Input 2"=w247:dbl[])  [unwired: 8 in]
            n81 = Index Array(array=w247) -> (element=w246:dbl)  [unwired: 1 in]
            n82 = Index Array(array=w252) -> (element #1=w251:string, element #2=w250:string)  [unwired: 2 in]
            n83 = Number To Fractional String(number=w246, precision (6)=i16 2) -> (F-format string=w253:string)  [unwired: 2 in]
            n84 = call <vilib>:"Trim Whitespace.vi"("string"=w251) -> ("trimmed string"=w272:string)  [unwired: 1 in]
            n85 = case shown="False" w277 {
              tunnel: w278 -> [w300 w334]
              tunnel: w248 -> [w302 w333]
              tunnel: [w308 w332] -> w275
              tunnel: [w307 w331] -> w270
              tunnel: w276 -> [w297 _]
              tunnel: w272 -> [w294 _]
              tunnel: w250 -> [w304 w324]
              tunnel: w253 -> [w288 _]
              frame False {
                w296 = string[] ["BARCODE", "SHIFT", "DATE", "ST1_LEAK_RATE", "ST1_FINAL_RST"]
                # "ST1 RESULT"
                # "DO TRACEBILITY"
                n86 = local read "SHIFT"() -> (w306:string)
                n87 = Format Into String(format string="Where BARCODE='%s' ", w294) -> (resulting string=w289:string)  [unwired: 2 in, 1 out]
                n88 = call <vilib>:"DB Tools Select Data.vi"("condition"=w289, "error in (no error)"=w302, "columns"=w296, "table"=w297, "connection reference"=w300) -> ("error out"=w298:errorcluster, "data"=w301:variant[][], "connection reference out"=w299:T13)  [unwired: 1 in]
                n89 = call "PADMINI_SHIFT_DATE.vi"("SHIFT"=w306) -> ("date/time string"=w305:string)  [unwired: 10 in]
                n90 = Variant To Data(error in=w298, type=string[][] [], Variant=w301) -> (data=w292:string[][], error out=w290:errorcluster)
                n91 = Bundle("trimmed string"=w294, "SHIFT"=w306, "date/time string"=w305, w288, "Input 2"=w304) -> (w303:T15)  [unwired: 1 in]
                n92 = Empty Array?(array=w292) -> (empty?=w291:bool)
                n93 = case shown="False" w291 {
                  tunnel: w299 -> [w313 w323]
                  tunnel: w290 -> [w312 w322]
                  tunnel: [w316 w321] -> w308
                  tunnel: [w315 w320] -> w307
                  tunnel: w296 -> [w310 w319]
                  tunnel: w297 -> [w311 w318]
                  tunnel: w303 -> [w314 w317]
                  tunnel: w289 -> [w309 _]
                  frame False {
                    n94 = call <vilib>:"DB Tools Update Data.vi"("condition"=w309, "data"=w314, "error in (no error)"=w312, "columns"=w310, "table"=w311, "connection reference"=w313) -> ("error out"=w315:errorcluster, "connection reference out"=w316:T13)  [unwired: 4 in]
                  }
                  frame True {
                    n95 = call <vilib>:"DB Tools Insert Data.vi"("data"=w317, "error in (no error)"=w322, "columns"=w319, "table"=w318, "connection reference"=w323) -> ("error out"=w320:errorcluster, "connection reference out"=w321:T13)  [unwired: 5 in]
                  }
                }
              }
              frame True {
                n96 = local read "SHIFT"() -> (w329:string)
                n97 = call "PADMINI_SHIFT_DATE.vi"("SHIFT"=w329) -> ("date/time string"=w328:string)  [unwired: 10 in]
                n98 = Bundle("SHIFT"=w329, "date/time string"=w328, "Input 2"=w324) -> (w327:T16)  [unwired: 1 in]
                n99 = To Variant(anything=w327) -> (Variant=w326:variant)
                n100 = call <vilib>:"DB Tools Insert Data.vi"("data"=w326, "error in (no error)"=w333, "columns"=string[] ["SHIFT", "DATE", "ST1_REAL_DATA", "ST1_BOOL_DATA", "ST1_RESULT", "RESULT"], "table"="ST1_REPORT", "connection reference"=w334) -> ("error out"=w331:errorcluster, "connection reference out"=w332:T13)  [unwired: 5 in]
              }
            }
            n101 = Bundle By Name(cluster=w256, "OP - 10.LEAK RATE"=w246) -> (w255:T11)
            n102 = call <vilib>:"Simple Error Handler.vi"("type of dialog (OK msg:1)"=w269, "error in (no error)"=w270) -> ("error out"=w268:errorcluster)  [unwired: 3 in, 4 out]
            n103 = call <vilib>:"Clear Errors.vi"("error in (no error)"=w268) -> ("error out"=w266:errorcluster)  [unwired: 5 in, 1 out]
            n104 = property on="OP - 10" class="Clust"(error in=w266) -> (error out=w260:errorcluster, "Controls[]"=w264:refnum<vi>[])  [unwired: 1 in, 1 out]
            n105 = Index Array(array=w264, index=2) -> (element=w262:refnum<vi>)
            n106 = To More Specific Class(target class=w261, reference=w262, error in=w260) -> (specific class reference=w265:refnum<vi>, error out=w259:errorcluster)
            n107 = call "PADMINI_BOOL_COLOR_CHANGE.vi"("error in (no error)"=w259, "Numeric"=w257, "Boolean in"=w265) -> ("error out"=w258:errorcluster)  [unwired: 8 in]
            n108 = disable-structure shown="Disabled" {
              disable-tunnel: [w281 w287] -> w274
              disable-tunnel: w258 -> [w280 w287]
              frame Disabled {
                n109 = call "PADMINI_AUTO_DATALOG_DONE.vi"("Enum"=enum16{"Read", "Write"}."Write", "error in (no error)"=w280, "I/P"=u16 2) -> ("error out"=w282:errorcluster)  [unwired: 7 in, 1 out]
                n110 = flat-sequence {
                  tunnel: [w285] -> w281
                  tunnel: w282 -> [w285]
                  frame #0 {
                    n111 = global write "DATA LOG.vi" "OP 10 DATA LOG RESULT"(TRUE ("DATA LOG RESET")) -> ()
                  }
                }
              }
              frame Enabled {
              }
            }
          }
          frame "SCAN2" {
            # "Barcode Status\n0-Ideal, 1-Ok, 2-Nok, 3-Prev Station Not Done,\n4-Prev Station Nok,\n5- Already Done"
            # "STATION OP 20"
            n112 = case shown="False" w341 {
              tunnel: w345 -> [w369 w403]
              tunnel: w344 -> [w361 w401]
              tunnel: w343 -> [_ _]
              tunnel: [w364 w400] -> w340
              tunnel: [w362 w403] -> w342
              frame False {
                # "2 FOR EMPTY BARCODE READ OR MISMATCH"
                n113 = call "PADMINI_AUTO_BARCODE_STRING2.vi"("Enum"=enum16{"Read", "Write"}."Read", "error in (no error)"=w361) -> ("error out"=w360:errorcluster, "Input 2"=w347:string[])  [unwired: 8 in]
                n114 = global read "Global 1.vi" "BARCODE RECIPE"() -> (w348:string)
                n115 = Index Array(array=w347) -> (element=w346:string)  [unwired: 1 in]
                n116 = call <vilib>:"Trim Whitespace.vi"("string"=w346) -> ("trimmed string"=w352:string)  [unwired: 1 in]
                n117 = Match Pattern(string=w352, regular expression=w348) -> (match substring=w349:string)  [unwired: 1 in, 3 out]
                n118 = String Length(string=w348) -> (length=w351:i32)
                n119 = String Length(string=w349) -> (length=w350:i32)
                n120 = Format Into String(format string="WHERE BARCODE  ='%s'", w352) -> (resulting string=w356:string)  [unwired: 2 in, 1 out]
                n121 = Equal?(x=w351, y=w350) -> (x = y?=w353:bool)
                n122 = call <vilib>:"DB Tools Select Data.vi"("condition"=w356, "error in (no error)"=w360, "columns"=string[] ["BARCODE", "ST1_FINAL_RST", "ST2_FINAL_RST"], "table"="REPORT", "connection reference"=w369) -> ("error out"=w367:errorcluster, "data"=w366:variant[][], "connection reference out"=w362:T13)  [unwired: 1 in]
                n123 = call "PADMINI_varient_to_data.vi"("error in (no error)"=w367, "data"=w366) -> ("error out"=w365:errorcluster, "Array"=w363:string[][])  [unwired: 8 in]
                n124 = Equal?(x=w352, y="") -> (x = y?=w354:bool)
                n125 = case shown="False" w354 {
                  selector: w354 -> [_ w398]
                  tunnel: w365 -> [w373 w397]
                  tunnel: [w372 w396] -> w364
                  tunnel: w363 -> [w371 _]
                  tunnel: w353 -> [w370 _]
                  frame False {
                    n126 = case shown="True" w370 {
                      tunnel: w373 -> [w376 w386]
                      tunnel: [w375 w393] -> w372
                      tunnel: w371 -> [_ w392]
                      frame False {
                        n127 = call "PADMINI_AUTO_BARCODE_STATUS 20.vi"("Enum"=enum16{"Read", "Write"}."Write", "error in (no error)"=w376, "I/P"=bool[] [FALSE, TRUE, FALSE, FALSE, FALSE, FALSE]) -> ("error out"=w375:errorcluster)  [unwired: 7 in, 1 out]
                      }
                      frame True {
                        # "ST2 RESULT"
                        # "ST1 RESULT"
                        n128 = Index Array(array=w392, index (row) #1=0 ("index (row)"), index (col) #1=1 ("disabled index (col)"), index (row) #2=0 ("index (row)"), index (col) #2=2 ("disabled index (col)")) -> (element #1=w385:string)  [unwired: 1 out]
                        n129 = Empty String/Path?(string/path=w385) -> (empty?=w383:bool)
                        n130 = Equal?(x=w385, y="OK") -> (x = y?=w379:bool)
                        n131 = Not(x=w379) -> (.not. x?=w378:bool)
                        n132 = Build Array(TRUE ("element"), FALSE ("element"), w383, w379, w378) -> (w382:bool[])
                        n133 = call "PADMINI_AUTO_BARCODE_STATUS 20.vi"("Enum"=enum16{"Read", "Write"}."Write", "error in (no error)"=w386, "I/P"=w382) -> ("error out"=w393:errorcluster)  [unwired: 7 in, 1 out]
                      }
                    }
                  }
                  frame True {
                    n134 = call "PADMINI_AUTO_BARCODE_STATUS 20.vi"("Enum"=enum16{"Read", "Write"}."Write", "error in (no error)"=w397, "I/P"=bool[] [FALSE, FALSE, FALSE, FALSE, FALSE]) -> ("error out"=w396:errorcluster)  [unwired: 7 in, 1 out]
                    "OP30 BARCODE STRING EMPRTY" <- w398
                  }
                }
              }
              frame True {
                n135 = call "PADMINI_AUTO_BARCODE_STATUS 20.vi"("Enum"=enum16{"Read", "Write"}."Write", "error in (no error)"=w401, "I/P"=bool[] [FALSE, FALSE, FALSE, FALSE, FALSE]) -> ("error out"=w400:errorcluster)  [unwired: 7 in, 1 out]
              }
            }
            n136 = flat-sequence {
              tunnel: [w406] -> w339
              tunnel: w340 -> [w406]
              frame #0 {
                # "UPDATE op 20 SCAN sTATUS"
                n137 = local write "OP30 BARCODE STRING EMPRTY"(FALSE ("Boolean 5")) -> ()
                n138 = global write "DATA LOG.vi" "OP 20 SCAN STATUS"(TRUE) -> ()
              }
            }
          }
          frame "DATALOG2" {
            w437 = T14 2 items=["no dialog", "OK message", "continue or stop message", "OK message + warnings", "continue/stop + warnings"] ("type of dialog (OK msg:1)")
            # "Printed QR Code data string"
            # "datalog of OP 20"
            n139 = call "PADMINI_AUTO_BARCODE_STRING2.vi"("Enum"=enum16{"Read", "Write"}."Read", "error in (no error)"=w424) -> ("error out"=w426:errorcluster, "Input 2"=w408:string[])  [unwired: 8 in]
            n140 = call "PADMINI_AUTO_CYCLE VALUE 20.vi"("Enum"=enum16{"Read", "Write"}."Read", "error in (no error)"=w424) -> ("Input 2"=w418:dbl[])  [unwired: 8 in, 1 out]
            n141 = Index Array(array=w418) -> (element #1=w423:dbl, element #2=w422:dbl, element #3=w421:dbl, element #4=w420:dbl)  [unwired: 4 in]
            n142 = Number To Fractional String(number=w418, precision (6)=i16 2) -> (F-format string=w417:string[])  [unwired: 2 in]
            n143 = case shown="False" w442 {
              tunnel: w443 -> [w478 w486]
              tunnel: w426 -> [w479 w485]
              tunnel: [w482 w484] -> w440
              tunnel: [w481 w483] -> w438
              tunnel: w441 -> [w477 _]
              tunnel: w417 -> [w473 _]
              tunnel: w408 -> [w465 _]
              frame False {
                # "ST2 RESULT"
                # "DO TRACEBILITY"
                n144 = Index Array(array=w465) -> (element #1=w466:string, element #2=w464:string, element #3=w463:string, element #4=w462:string, element #5=w461:string, element #6=w460:string, element #7=w459:string)  [unwired: 7 in]
                n145 = local read "SHIFT"() -> (w480:string)
                n146 = Index Array(array=w473) -> (element #1=w472:string, element #2=w471:string, element #3=w470:string, element #4=w469:string)  [unwired: 4 in]
                n147 = call <vilib>:"Trim Whitespace.vi"("string"=w466) -> ("trimmed string"=w467:string)  [unwired: 1 in]
                n148 = call "PADMINI_SHIFT_DATE.vi"("SHIFT"=w480) -> ()  [unwired: 10 in, 1 out]
                n149 = Format Into String(format string="Where BARCODE='%s' ", w467) -> (resulting string=w475:string)  [unwired: 2 in, 1 out]
                n150 = Bundle("Input 2"=w472, "Input 2"=w471, "Input 2"=w464, "Input 2"=w463, "Input 2"=w470, "Input 2"=w469, "Input 2"=w462, "Input 2"=w461, "Input 2"=w460, "Input 2"=w459) -> (w468:T17)  [unwired: 1 in]
                n151 = call <vilib>:"DB Tools Update Data.vi"("condition"=w475, "data"=w468, "error in (no error)"=w479, "columns"=string[] ["ST2_LOWER_BEARING_DIS", "ST2_LOWER_BEARING_LOAD", "ST2_BOTTOM_CAMERA_STATUS", "ST2_LOWER_BEARING_RST", "ST2_UPPER_BEARING_DIS", "ST2_UPPER_BEARING_LOAD", "ST2_UPPER_SIM_STATUS", "ST2_UPPER_CAMERA_STATUS", "ST2_UPPER_BERAING_RST", "ST2_FINAL_RST"], "table"=w477, "connection reference"=w478) -> ("error out"=w481:errorcluster, "connection reference out"=w482:T13)  [unwired: 4 in]
              }
              frame True {
                n152 = disable-structure shown="Disabled" {
                  disable-tunnel: w486 -> [w496 _]
                  disable-tunnel: w485 -> [w495 _]
                  disable-tunnel: [w494 _] -> w484
                  disable-tunnel: [w493 _] -> w483
                  frame Disabled {
                    n153 = local read "SHIFT"() -> (w491:string)
                    n154 = call "PADMINI_SHIFT_DATE.vi"("SHIFT"=w491) -> ("date/time string"=w490:string)  [unwired: 10 in]
                    n155 = Bundle("SHIFT"=w491, "date/time string"=w490) -> (w489:T18)  [unwired: 2 in]
                    n156 = To Variant(anything=w489) -> (Variant=w488:variant)
                    n157 = call <vilib>:"DB Tools Insert Data.vi"("data"=w488, "error in (no error)"=w495, "columns"=string[] ["SHIFT", "DATE", "ST1_REAL_DATA", "ST1_BOOL_DATA", "ST1_RESULT", "RESULT"], "table"="ST1_REPORT", "connection reference"=w496) -> ("error out"=w493:errorcluster, "connection reference out"=w494:T13)  [unwired: 5 in]
                  }
                  frame Enabled {
                  }
                }
              }
            }
            n158 = Bundle By Name(cluster=w429, "OP - 20.LOWERING BEARING DISPLACE"=w423, "OP - 20.LOWERING BEARING LOAD"=w422, "OP - 20.UPPER BEARING DISPLACE"=w421, "OP - 20.UPPER BEARING LOAD"=w420) -> (w428:T11)
            n159 = call <vilib>:"Simple Error Handler.vi"("type of dialog (OK msg:1)"=w437, "error in (no error)"=w438) -> ("error out"=w436:errorcluster)  [unwired: 3 in, 4 out]
            n160 = call <vilib>:"Clear Errors.vi"("error in (no error)"=w436) -> ("error out"=w434:errorcluster)  [unwired: 5 in, 1 out]
            n161 = property on="OP - 20" class="Clust"(error in=w434) -> (error out=w431:errorcluster, "Controls[]"=w433:refnum<vi>[])  [unwired: 1 in, 1 out]
            n162 = for {
              tunnel: w408 -> [w448] mode=indexing
              tunnel: [w447] -> w407 mode=indexing if=w445
              i -> [w446]
              n163 = case shown="\"NG\"" w448 {
                tunnel: [2 ("CYCLE STATUS OK, NOK, ABORTED") 1 ("CYCLE STATUS OK, NOK, ABORTED") 0 ("CYCLE STATUS OK, NOK, ABORTED")] -> w447
                frame "NG" {
                }
                frame "OK" {
                }
                frame "-1", Default {
                }
              }
              n164 = Not Equal To 0?(x=w446) -> (x != 0?=w445:bool)
            }
            n165 = Index Array(array=w433, index #1=3 ("index"), index #3=7 ("index")) -> (element #1=w415:refnum<vi>, element #2=w414:refnum<vi>, element #3=w413:refnum<vi>, element #4=w412:refnum<vi>, element #5=w411:refnum<vi>, element #6=w410:refnum<vi>)  [unwired: 4 in]
            n166 = Build Array(w415, w414, w413, w412, w411, w410) -> (w409:refnum<vi>[])
            n167 = for {
              tunnel: w409 -> [w457] mode=indexing
              shift-right: [w453] -> w430
              shift-left: w431 -> [w455]
              tunnel: w407 -> [w452] mode=indexing
              w456 = refnum<vi> refnum  # Boolean
              n168 = To More Specific Class(target class=w456, reference=w457, error in=w455) -> (specific class reference=w458:refnum<vi>, error out=w454:errorcluster)
              n169 = call "PADMINI_BOOL_COLOR_CHANGE.vi"("error in (no error)"=w454, "Numeric"=w452, "Boolean in"=w458) -> ("error out"=w453:errorcluster)  [unwired: 8 in]
            }
          }
          frame "SCAN3" {
            n170 = case shown="False" w502 {
              tunnel: w506 -> [w530 w620]
              tunnel: w505 -> [w529 w618]
              tunnel: w504 -> [w528 _]
              tunnel: [w519 w617] -> w501
              tunnel: [w522 w620] -> w503
              frame False {
                # "Barcode Status\n0-Ideal, 1-Ok, 2-Nok, 3-Prev Station Not Done,\n4-Prev Station Nok,\n5- Already Done"
                # "0 = IF STATION 1 RESULT IS EMPTY\n1 = IF STATION 1 RESULT IS TRUE IS (LOGGED)\n       AND STATION 2 RESULT IS EMPTY (NOT LOGGED YET)\n2 = IF STATION 1 DATA IS LODDED BUT ITS FALSE(NOK)\n3 = IF STATION 2 RESULT IS STILL EMPTY ( YET NOT LOGGED)"
                n171 = global read "DATA LOG.vi" "ST 3 STRING 2"() -> (w517:string)
                n172 = call <vilib>:"Trim Whitespace.vi"("string"=w517) -> ("trimmed string"=w514:string)  [unwired: 1 in]
                n173 = disable-structure shown="Enabled" {
                  disable-tunnel: w514 -> [w532 _]
                  disable-tunnel: [w533 TRUE] -> w513
                  frame Enabled {
                    (unwired) "False"
                    (unwired) "True"
                    n174 = global read "Global 1.vi" "BARCODE RECIPE"() -> (w531:string)
                    n175 = Match Pattern(string=w532, regular expression=w531) -> (match substring=w536:string)  [unwired: 1 in, 3 out]
                    n176 = String Length(string=w531) -> (length=w535:i32)
                    n177 = String Length(string=w536) -> (length=w534:i32)
                    n178 = Equal?(x=w535, y=w534) -> (x = y?=w533:bool)
                  }
                  frame Disabled {
                  }
                }
                n179 = Format Into String(format string="where BARCODE='%s'", w514) -> (resulting string=w525:string)  [unwired: 2 in, 1 out]
                n180 = call <vilib>:"DB Tools Select Data.vi"("condition"=w525, "error in (no error)"=w529, "columns"=string[] ["BARCODE", "ST2_RESULT", "ST3_RESULT"], "table"=w528, "connection reference"=w530) -> ("error out"=w524:errorcluster, "data"=w523:variant[][], "connection reference out"=w522:T13)  [unwired: 1 in]
                n181 = Equal?(x=w514, y="") -> (x = y?=w515:bool)
                n182 = case shown="False" w515 {
                  selector: w515 -> [_ w615]
                  tunnel: w524 -> [w542 w613]
                  tunnel: w523 -> [w541 _]
                  tunnel: [w540 w613] -> w520
                  tunnel: [w539 2] -> w518
                  tunnel: w513 -> [w538 _]
                  frame False {
                    n183 = case shown="True" w538 {
                      tunnel: w542 -> [w543 w579]
                      tunnel: w541 -> [_ w578]
                      tunnel: [w543 w569] -> w540
                      tunnel: [u16 2 ("I/P") w568] -> w539
                      frame False {
                      }
                      frame True {
                        (unwired) "OK"
                        (unwired) "OK"
                        n184 = call "PADMINI_varient_to_data.vi"("error in (no error)"=w579, "data"=w578) -> ("error out"=w550:errorcluster, "Array"=w570:string[][])  [unwired: 8 in]
                        n185 = Index Array(array=w570, index (row) #1=0 ("index (row)"), index (col) #1=1 ("disabled index (col)"), index (row) #2=0 ("index (row)"), index (col) #2=2 ("disabled index (col)")) -> (element #1=w553:string, element #2=w547:string)
                        n186 = call <vilib>:"Clear Errors.vi"("error in (no error)"=w550) -> ("error out"=w549:errorcluster)  [unwired: 5 in, 1 out]
                        n187 = Not Equal?(x=w553, y="OK") -> (x != y?=w576:bool)
                        n188 = Equal?(x=w553, y="OK") -> (x = y?=w555:bool)
                        n189 = Empty String/Path?(string/path=w553) -> (empty?=w577:bool)
                        n190 = Empty String/Path?(string/path=w547) -> (empty?=w571:bool)
                        n191 = call "RECHECK READ BIT.vi"("Enum"=enum16{"Read", "Write"}."Read", "error in (no error)"=w549) -> ("error out"=w556:errorcluster, "Input 2"=w560:dbl[])  [unwired: 8 in]
                        n192 = Equal?(x=w547, y="Aborted") -> (x = y?=w545:bool)
                        n193 = Equal?(x=w547, y="NOK") -> (x = y?=w546:bool)
                        n194 = And(x=w555, y=w571) -> (x .and. y?=w572:bool)
                        n195 = Not(x=w571) -> (.not. x?=w567:bool)
                        n196 = Index Array(array=w560, index=0) -> (element=w561:dbl)
                        n197 = Build Array(w577, w572, w576, w567) -> (w575:bool[])
                        n198 = Equal?(x=w561, y=1.0) -> (x = y?=w551:bool)
                        n199 = Search 1D Array(1D array=w575, element=TRUE) -> (index of element=w573:i32)  [unwired: 1 in]
                        n200 = case shown="True" w551 {
                          tunnel: w573 -> [w583 _]
                          tunnel: [w582 w595] -> w569
                          tunnel: [w581 w598] -> w568
                          tunnel: w556 -> [w580 w596]
                          tunnel: w546 -> [_ w597]
                          tunnel: w545 -> [_ w594]
                          frame False {
                            n201 = case shown="3" w583 {
                              tunnel: [w585 w586 w588 w590 w593] -> w582
                              tunnel: w580 -> [w585 w586 w588 w590 w593]
                              tunnel: [u16 0 ("I/P") u16 3 ("I/P") u16 1 ("I/P") u16 4 ("I/P") u16 5 ("I/P")] -> w581
                              frame -1, Default {
                              }
                              frame 0 {
                              }
                              frame 1 {
                              }
                              frame 2 {
                              }
                              frame 3 {
                              }
                            }
                          }
                          frame True {
                            n202 = case shown="False" w597 {
                              tunnel: [w602 u16 1 ("I/P")] -> w598
                              tunnel: w596 -> [w601 w611]
                              tunnel: [w600 w611] -> w595
                              tunnel: w594 -> [w599 _]
                              frame False {
                                n203 = case shown="False" w599 {
                                tunnel: [u16 5 ("I/P") u16 1 ("I/P")] -> w602
                                tunnel: w601 -> [w604 w610]
                                tunnel: [w603 w610] -> w600
                                frame False {
                                n204 = global write "Global 1.vi" "RECHECK RESULT OK"(TRUE ("RECHECK RESULT OK")) -> ()
                                n205 = call "SEND RECHECK ABORT BUTTON.vi"("Enum"=enum16{"Read", "Write"}."Write", "error in (no error)"=w604, "Array"=u16[] [0]) -> ("error out"=w603:errorcluster)  [unwired: 7 in, 1 out]
                                }
                                frame True {
                                }
                                }
                              }
                              frame True {
                              }
                            }
                          }
                        }
                      }
                    }
                  }
                  frame True {
                    "OP40 BARCODE STRING EMPRTY" <- w615
                  }
                }
                n206 = call "PADMINI_AUTO_BARCODE_STATUS3.vi"("Enum"=enum16{"Read", "Write"}."Write", "error in (no error)"=w520, "I/P"=w518) -> ("error out"=w519:errorcluster)  [unwired: 7 in, 1 out]
              }
              frame True {
                n207 = call "PADMINI_AUTO_BARCODE_STATUS3.vi"("Enum"=enum16{"Read", "Write"}."Write", "error in (no error)"=w618, "I/P"=u16 1) -> ("error out"=w617:errorcluster)  [unwired: 7 in, 1 out]
              }
            }
            n208 = flat-sequence {
              tunnel: [w512] -> w500
              tunnel: w501 -> [w512]
              frame #0 {
                n209 = local write "OP40 BARCODE STRING EMPRTY"(FALSE) -> ()
                n210 = global write "DATA LOG.vi" "scan op 40"(TRUE ("scan op 40")) -> ()
                n211 = global write "DATA LOG.vi" "ST 3 STRING 2"("" ("ST 3 STRING 2")) -> ()
                n212 = global write "DATA LOG.vi" "op 40"(0 ("op 30")) -> ()
              }
            }
          }
          frame "EMERGENCY STOP" {
          }
          frame "STOP" {
            n213 = global read "Global 1.vi" "BARCODE RECIPE"() -> (w631:string)
            n214 = Bundle("BARCODE RECIPE"=w631) -> (w630:cluster{"BARCODE RECIPE":string})  [unwired: 1 in]
            n215 = call <vilib>:"DB Tools Update Data.vi"("data"=w630, "error in (no error)"=w636, "columns"=string[] ["PREVIOUS_LOADED_RECIPE"], "table"="BARCODE_RECIPE", "connection reference"=w634) -> ("error out"=w635:errorcluster, "connection reference out"=w633:T13)  [unwired: 5 in]
          }
        }
      }
      frame Error {
        # "Return true in any case that should stop the loop."
      }
    }
    n216 = Unbundle By Name(w123) -> ("OP - 90"=→"OP - 90":T8, "OP - 100"=→"OP - 100":T9, "OP - 110"=→"OP - 110":cluster{"BARCODE":string})
    n217 = Unbundle By Name(w123) -> ("OP - 10"=→"OP - 10":T4, "OP - 20"=→"OP - 20":T19, "OP - 30"=→"OP - 30":T3, "OP - 40"=→"OP - 40":T2)
    n218 = Unbundle By Name(w123) -> ("OP - 50"=→"OP - 50":T1, "OP - 60"=→"OP - 60":T10, "OP - 70"=→"OP - 70":T7, "OP - 80"=→"OP - 80":T6)
    n219 = Wait (ms)(milliseconds to wait=u32 100) -> ()  [unwired: 1 out]
  }
  n220 = while {
    shift-right: [w671] -> w71
    shift-left: w20 -> [w665]
    shift-right: [w672] -> w65
    shift-left: w69 -> [w680]
    stop <- w670 stop-if-true
    w649 = enum16{"Read", "Write"}."Read" ("Enum")
    n221 = local read "Shift_change"() -> (w678:bool)
    n222 = call <vilib>:"Clear Errors.vi"("error in (no error)"=w665) -> ("error out"=w648:errorcluster)  [unwired: 5 in, 1 out]
    n223 = call "READ EMERGENCY BIT.vi"("Enum"=enum16{"Read", "Write"}."Read", "error in (no error)"=w648) -> ("Array Out"=w668:dbl[])  [unwired: 8 in, 1 out]
    n224 = case shown="True" w678 {
      tunnel: w648 -> [w703 w716]
      tunnel: [w704 w715] -> w677
      frame False {
        n225 = local read "SHIFT_DATA 2"() -> (w706:string[])
        n226 = Get Date/Time In Seconds() -> (seconds since 1Jan1904=w705:timestamp)
        n227 = call "String To Time_4.vi"("error in (no error)"=w703, "String Array In"=w706) -> ("error out"=w702:errorcluster, "Time Stamp Out"=w701:timestamp[])  [unwired: 8 in]
        "Time Stamp Out 4" <- w701
        n228 = call "Shift Calculation_4.vi"("error in (no error)"=w702, "Current Time"=w705, "Time Stamp Out"=w701) -> ("error out"=w700:errorcluster, "Shift"=w699:i32)  [unwired: 7 in]
        n229 = call <vilib>:"Clear Errors.vi"("error in (no error)"=w700) -> ()  [unwired: 5 in, 2 out]
        n230 = case shown="4" w699 {
          tunnel: ["A" "B" "C" "D"] -> w704
          frame 1, Default {
          }
          frame 2 {
          }
          frame 3 {
          }
          frame 4 {
          }
        }
      }
      frame True {
        n231 = local read "SHIFT_DATA"() -> (w714:string[])
        n232 = Get Date/Time In Seconds() -> (seconds since 1Jan1904=w717:timestamp)
        n233 = call "String To Time.vi"("error in (no error)"=w716, "String Array In"=w714) -> ("error out"=w713:errorcluster, "Time Stamp Out"=w718:timestamp[])  [unwired: 8 in]
        "Time Stamp Out" <- w718
        n234 = call "Shift Calculation.vi"("error in (no error)"=w713, "Current Time"=w717, "Time Stamp Out"=w718) -> ("error out"=w712:errorcluster, "Shift"=w711:i32)  [unwired: 7 in]
        "Shift 4" <- w711
        n235 = call <vilib>:"Clear Errors.vi"("error in (no error)"=w712) -> ()  [unwired: 5 in, 2 out]
        n236 = case shown="3" w711 {
          tunnel: ["A" "B" "C"] -> w715
          frame 1, Default {
          }
          frame 2 {
          }
          frame 3 {
          }
        }
      }
    }
    "SHIFT" <- w677
    n237 = call "PADMINI_AUTO_CYCLE STATE 30.vi"("Enum"=w649, "error in (no error)"=w648) -> ("error out"=w647:errorcluster, "Input 2"=w646:bool[])  [unwired: 8 in]
    n238 = call "PADMINI_AUTO_CYCLE STATE 20.vi"("Enum"=w649, "error in (no error)"=w648) -> ("error out"=w660:errorcluster, "Input 2"=w657:bool[])  [unwired: 8 in]
    n239 = call "PADMINI_AUTO_CYCLE STATE.vi"("Enum"=w649, "error in (no error)"=w648) -> ("error out"=w659:errorcluster, "Input 2"=w655:bool[])  [unwired: 8 in]
    n240 = Index Array(array=w668) -> (element=w667:dbl)  [unwired: 1 in]
    n241 = Merge Errors(w659, w660, w647) -> (w658:errorcluster)
    n242 = call "VALUE_CHANGE - ST1_RESULT.vi"("Numeric"=w667) -> ("Boolean"=w666:bool)  [unwired: 9 in, 1 out]
    n243 = global write "Global 1.vi" "EMERGENCY STOP"(w666) -> ()
    n244 = for {
      tunnel: w655 -> [w685] mode=indexing
      tunnel: [w684] -> w654 mode=indexing
      n245 = call <userlib>:"Boolean Trigger__ogtk.vi"("Boolean Input"=w685) -> ("Rising Edge"=w684:bool)  [unwired: 1 in, 1 out]
    }
    n246 = for {
      tunnel: w657 -> [w687] mode=indexing
      tunnel: [w686] -> w656 mode=indexing
      n247 = call <userlib>:"Boolean Trigger__ogtk.vi"("Boolean Input"=w687) -> ("Rising Edge"=w686:bool)  [unwired: 1 in, 1 out]
    }
    n248 = for {
      tunnel: w646 -> [w683] mode=indexing
      tunnel: [w682] -> w645 mode=indexing
      n249 = call <userlib>:"Boolean Trigger__ogtk.vi"("Boolean Input"=w683) -> ("Rising Edge"=w682:bool)  [unwired: 1 in, 1 out]
    }
    n250 = Build Array (concatenate)(w654, w656, w645) -> (w661:bool[])
    n251 = for {
      tunnel: w661 -> [w842] mode=indexing
      tunnel: [w843] -> w681 mode=indexing if=w842
      i -> [w843]
    }
    n252 = for {
      tunnel: w681 -> [w722] mode=indexing
      shift-right: [w726] -> w674
      shift-left: w680 -> [w725]
      shift-right: [w724] -> w673
      shift-left: w658 -> [w723]
      n253 = case shown="5" w722 {
        tunnel: [w728 w734 w739 w744 w749 w754 w759 w764 w769 w774 w779 w784 w789 w794 w799 w804 w809 w814 w819 w824 w829 w834 w839] -> w726
        tunnel: w725 -> [w730 w736 w741 w746 w751 w756 w761 w766 w771 w776 w781 w786 w791 w796 w801 w806 w811 w816 w821 w826 w831 w836 w841]
        tunnel: [w727 w733 w738 w743 w748 w753 w758 w763 w768 w773 w778 w783 w788 w793 w798 w803 w808 w813 w818 w823 w828 w833 w838] -> w724
        tunnel: w723 -> [w729 w735 w740 w745 w750 w755 w760 w765 w770 w775 w780 w785 w790 w795 w800 w805 w810 w815 w820 w825 w830 w835 w840]
        frame -1, Default {
          # "DEFAULT"
          n254 = Enqueue Element(queue=w730, element=cluster{"CASE":T12} {"CASE"=enum."-1"}, error in (no error)=w729) -> (queue out=w728:refnum<queue>, error out=w727:errorcluster)  [unwired: 1 in, 1 out]
        }
        frame 0 {
          # "SCAN BARCODE OP 10"
          n255 = Enqueue Element(queue=w736, element=cluster{"CASE":T12} {"CASE"=enum."SCAN1"}, error in (no error)=w735) -> (queue out=w734:refnum<queue>, error out=w733:errorcluster)  [unwired: 1 in, 1 out]
        }
        frame 1 {
          # "DATALOG OF OP 10"
          n256 = Enqueue Element(queue=w741, element=cluster{"CASE":T12} {"CASE"=enum."DATALOG1"}, error in (no error)=w740) -> (queue out=w739:refnum<queue>, error out=w738:errorcluster)  [unwired: 1 in, 1 out]
        }
        frame 2 {
          # "SCAN BARCODE OP 20"
          n257 = Enqueue Element(queue=w746, element=cluster{"CASE":T12} {"CASE"=enum."SCAN2"}, error in (no error)=w745) -> (queue out=w744:refnum<queue>, error out=w743:errorcluster)  [unwired: 1 in, 1 out]
        }
        frame 3 {
          # "DATALOG OF OP 20"
          n258 = Enqueue Element(queue=w751, element=cluster{"CASE":T12} {"CASE"=enum."DATALOG2"}, error in (no error)=w750) -> (queue out=w749:refnum<queue>, error out=w748:errorcluster)  [unwired: 1 in, 1 out]
        }
        frame 4 {
          # "SCAN BARCODE OP 30"
          n259 = Enqueue Element(queue=w756, element=cluster{"CASE":T12} {"CASE"=enum."SCAN3"}, error in (no error)=w755) -> (queue out=w754:refnum<queue>, error out=w753:errorcluster)  [unwired: 1 in, 1 out]
        }
        frame 5 {
          # "DATALOG OF OP 30"
          n260 = Enqueue Element(queue=w761, element=cluster{"CASE":T12} {"CASE"=enum."DATALOG3"}, error in (no error)=w760) -> (queue out=w759:refnum<queue>, error out=w758:errorcluster)  [unwired: 1 in, 1 out]
        }
        frame 6 {
          # "SCAN BARCODE OP 40"
          n261 = Enqueue Element(queue=w766, element=cluster{"CASE":T12} {"CASE"=enum."SCAN4"}, error in (no error)=w765) -> (queue out=w764:refnum<queue>, error out=w763:errorcluster)  [unwired: 1 in, 1 out]
        }
        frame 7 {
          # "DATALOG OF OP 40"
          n262 = Enqueue Element(queue=w771, element=cluster{"CASE":T12} {"CASE"=enum."DATALOG4"}, error in (no error)=w770) -> (queue out=w769:refnum<queue>, error out=w768:errorcluster)  [unwired: 1 in, 1 out]
        }
        frame 8 {
          # "SCAN BARCODE OP 50"
          n263 = Enqueue Element(queue=w776, element=cluster{"CASE":T12} {"CASE"=enum."SCAN5"}, error in (no error)=w775) -> (queue out=w774:refnum<queue>, error out=w773:errorcluster)  [unwired: 1 in, 1 out]
        }
        frame 9 {
          # "DATALOG OF OP 50"
          n264 = Enqueue Element(queue=w781, element=cluster{"CASE":T12} {"CASE"=enum."DATALOG5"}, error in (no error)=w780) -> (queue out=w779:refnum<queue>, error out=w778:errorcluster)  [unwired: 1 in, 1 out]
        }
        frame 10 {
          # "SCAN BARCODE OP 60"
          n265 = Enqueue Element(queue=w786, element=cluster{"CASE":T12} {"CASE"=enum."SCAN6"}, error in (no error)=w785) -> (queue out=w784:refnum<queue>, error out=w783:errorcluster)  [unwired: 1 in, 1 out]
        }
        frame 11 {
          # "DATALOG OF OP 60"
          n266 = Enqueue Element(queue=w791, element=cluster{"CASE":T12} {"CASE"=enum."DATALOG6"}, error in (no error)=w790) -> (queue out=w789:refnum<queue>, error out=w788:errorcluster)  [unwired: 1 in, 1 out]
        }
        frame 12 {
          # "SCAN BARCODE OP 70"
          n267 = Enqueue Element(queue=w796, element=cluster{"CASE":T12} {"CASE"=enum."SCAN7"}, error in (no error)=w795) -> (queue out=w794:refnum<queue>, error out=w793:errorcluster)  [unwired: 1 in, 1 out]
        }
        frame 13 {
          # "DATALOG OF OP 70"
          n268 = Enqueue Element(queue=w801, element=cluster{"CASE":T12} {"CASE"=enum."DATALOG7"}, error in (no error)=w800) -> (queue out=w799:refnum<queue>, error out=w798:errorcluster)  [unwired: 1 in, 1 out]
        }
        frame 14 {
          # "SCAN BARCODE 80"
          n269 = Enqueue Element(queue=w806, element=cluster{"CASE":T12} {"CASE"=enum."SCAN8"}, error in (no error)=w805) -> (queue out=w804:refnum<queue>, error out=w803:errorcluster)  [unwired: 1 in, 1 out]
        }
        frame 15 {
          # "DATALOG OF OP 80"
          n270 = Enqueue Element(queue=w811, element=cluster{"CASE":T12} {"CASE"=enum."DATALOG8"}, error in (no error)=w810) -> (queue out=w809:refnum<queue>, error out=w808:errorcluster)  [unwired: 1 in, 1 out]
        }
        frame 16 {
          # "SCAN BARCODE OP 90"
          n271 = Enqueue Element(queue=w816, element=cluster{"CASE":T12} {"CASE"=enum."SCAN9"}, error in (no error)=w815) -> (queue out=w814:refnum<queue>, error out=w813:errorcluster)  [unwired: 1 in, 1 out]
        }
        frame 17 {
          # "DATALOG OF OP 90"
          n272 = Enqueue Element(queue=w821, element=cluster{"CASE":T12} {"CASE"=enum."DATALOG9"}, error in (no error)=w820) -> (queue out=w819:refnum<queue>, error out=w818:errorcluster)  [unwired: 1 in, 1 out]
        }
        frame 18 {
          # "SCAN BARCODE OP 100"
          n273 = Enqueue Element(queue=w826, element=cluster{"CASE":T12} {"CASE"=enum."SCAN10"}, error in (no error)=w825) -> (queue out=w824:refnum<queue>, error out=w823:errorcluster)  [unwired: 1 in, 1 out]
        }
        frame 19 {
          # "DATALOG OF OP 100"
          n274 = Enqueue Element(queue=w831, element=cluster{"CASE":T12} {"CASE"=enum."DATALOG10"}, error in (no error)=w830) -> (queue out=w829:refnum<queue>, error out=w828:errorcluster)  [unwired: 1 in, 1 out]
        }
        frame 20 {
          # "SCAN BARCODE OP 110"
          n275 = Enqueue Element(queue=w836, element=cluster{"CASE":T12} {"CASE"=enum."SCAN11"}, error in (no error)=w835) -> (queue out=w834:refnum<queue>, error out=w833:errorcluster)  [unwired: 1 in, 1 out]
        }
        frame 21 {
          # "DATALOG OF OP 110"
          n276 = Enqueue Element(queue=w841, element=cluster{"CASE":T12} {"CASE"=enum."DATALOG11"}, error in (no error)=w840) -> (queue out=w839:refnum<queue>, error out=w838:errorcluster)  [unwired: 1 in, 1 out]
        }
      }
    }
    n277 = Wait (ms)(milliseconds to wait=u32 50) -> ()  [unwired: 1 out]
    n278 = global read "Global 1.vi" "PLC COMM"() -> (→"PLC COM.":bool)
    n279 = global read "Global 1.vi" "PLC 1"() -> (→"OP 10 & 20":bool)
    n280 = global read "Global 1.vi" "PLC 2"() -> (→"OP 30":bool)
    n281 = global read "Global 1.vi" "PLC 3"() -> (→"OP 40":bool)
    n282 = case shown="True" "stop 2" {
      tunnel: w674 -> [w690 w696]
      tunnel: [w690 w695] -> w672
      tunnel: w673 -> [w689 w694]
      tunnel: [w689 w693] -> w671
      tunnel: [FALSE TRUE] -> w670
      frame False {
      }
      frame True {
        n283 = Flush Queue(queue=w696, error in (no error)=w694) -> (queue out=w698:refnum<queue>, error out=w697:errorcluster)  [unwired: 1 out]
        n284 = Enqueue Element(queue=w698, element=cluster{"CASE":T12} {"CASE"=enum."STOP"}, error in (no error)=w697) -> (queue out=w695:refnum<queue>, error out=w693:errorcluster)  [unwired: 1 in, 1 out]
      }
    }
    "stop" <- w670
    n285 = global read "Global 1.vi" "PLC 4"() -> (→"OP 50":bool)
    n286 = global read "Global 1.vi" "PLC 5"() -> (→"OP 60":bool)
    n287 = global read "Global 1.vi" "PLC 7"() -> (→"OP 90 -100 - 110":bool)
    n288 = global read "Global 1.vi" "PLC 6"() -> (→"OP 70 & 80":bool)
  }
  n289 = Release Queue(queue=w65, error in (no error)=w71) -> (error out=w48:errorcluster)  [unwired: 1 in, 2 out]
  n290 = call <vilib>:"Clear Errors.vi"("error in (no error)"=w67) -> ("error out"=w52:errorcluster)  [unwired: 5 in, 1 out]
  n291 = call <vilib>:"DB Tools Close Connection.vi"("error in (no error)"=w52, "connection reference"=w66) -> ("error out"=w49:errorcluster)  [unwired: 5 in]
  n292 = Merge Errors(w48, w49) -> (w50:errorcluster)
  n293 = call <vilib>:"Simple Error Handler.vi"("error in (no error)"=w50) -> ("error out"=w45:errorcluster)  [unwired: 4 in, 4 out]
  n294 = call <vilib>:"Clear Errors.vi"("error in (no error)"=w45) -> ("error out"=w51:errorcluster)  [unwired: 5 in, 1 out]
  n295 = flat-sequence {
    tunnel: w51 -> [w845]
    tunnel: [w845] -> w53
    frame #0 {
      n296 = global write "Global 1.vi" "REMOVE VI"(TRUE ("remove_VI")) -> ()
    }
  }
  n297 = property class="App"(error in=w53) -> (error out=w55:errorcluster, "App.Kind"=w54:T20)  [unwired: 1 in, 1 out]
  n298 = case shown="\"Run Time System\"" w54 {
    tunnel: [w846 w848] -> w56
    tunnel: w55 -> [w846 w847]
    frame "Development System", Default {
    }
    frame "Run Time System" {
      n299 = invoke class="VI" method="FP.Close"(error in=w847) -> (error out=w848:errorcluster)  [unwired: 2 in, 2 out]
    }
  }
  "error out 2" <- w56
